vi "coke_can_current_version.vi"() -> ()   [LabVIEW 2012]
uses:
  X:/Lab/Labmembers/Lukas Gemar/Control 1.ctl
  <vilib>/DAQmx/write.llb/DAQmx Write (Digital Bool 1Line 1Point).vi
  <vilib>/Analysis/baseanly.llb/Mean (DBL).vi
  <vilib>/DAQmx/create/channels.llb/DAQmx Create Channel (DO-Digital Output).vi
  <vilib>/DAQmx/miscellaneous.llb/DAQmx Fill In Error Info.vi
  <vilib>/Analysis/NI_AALBase.lvlib
  Program Files/ALP-4.1/ALP-4.1 high-speed API/Samples/alpD41.dll
panel:
  in  "Bin (n x n) 2":u16(ring)=1 caption="Cursor Bin" items=["1x1"=1, "2x2"=2, "4x4"=4]
  in  "Tab Control":T1(tab)
  out "Initialize":u32
  out "Initialize?":bool
  out "Bits per Channel":i32
  out "camera initialization error":errorcluster
  out "Camera ID":string="0"
  out "Model":string="0"
  out "y pixels":i32
  out "x pixels":i32
  out "ROI cursor":T2={"x offset"=480, "y offset"=456, "x width"=68, "y width"=76} {"x offset" min=1 max=512 step=1; "y offset" min=1 max=512 step=1; "x width" min=1 max=512 step=1; "y width" min=1 max=512 step=1}
  out "Previous Bin":u16(ring)=2 caption="Cursor Bin" items=["1x1"=1, "2x2"=2, "4x4"=4]
  in  "473nm line":tag="Dev1/ao1"
  in  "635nm dig line":tag="Dev1/port0/line2"
  out "SerialNumber":i32
  out "DevAllocErr":i32
  out "DevInq1":errorcluster
  in  "Select Mov":bool
  in  "User Movie Path":path=path "C:/data/Lukas_data/movie.bin"
  in  "635nm":bool
  in  "All On":bool
  out "Movie Complete":bool caption="Movie Complete:"
  in  "Play Movie":bool
  in  "Make Movie":bool
  in  "Define Object":bool
  in  "Previous ROI 2":bool
  out "Previous ROI":T2={"x offset"=256, "y offset"=256, "x width"=512, "y width"=512} caption="Previous" {"x offset" min=1 max=512 step=1; "y offset" min=1 max=512 step=1; "x width" min=1 max=512 step=1; "y width" min=1 max=512 step=1}
  in  "Update ROI":bool
  in  "ROI":T2={"x offset"=960, "y offset"=912, "x width"=136, "y width"=152} caption="Current" {"x offset" min=1 max=2048 step=1; "y offset" min=1 max=2048 step=1; "x width" min=1 max=2048 step=1; "y width" min=1 max=2048 step=1}
  in  "Symmetrical":bool=TRUE
  in  "Draw ROI":bool
  in  "ROI selection":u16(ring) items=["Full ROI", "Central quad", "Red Laser ROI", "Custom ROI"]
  in  "Stop Program":bool
  in  "Enter Live Mode":bool
  out "Image":i32[][](graph)
  out "mean":dbl=701.2764784557547
  out "max value":u16=1056
  out "min value":u16=384
  out "Histogram":T3(graph)={"X Values"=[417.6, 484.8, 552.0, 619.2, 686.4, 753.6, 820.8, 888.0, 955.2, 1022.4], "Histogram: h(x)"=[403, 4234, 6440, 8496, 9541, 10568, 10361, 4568, 669, 48]}
  out "Camera Error":errorcluster
  out "Location indicator":u16[][](graph)
  in  "Clicky Movie Path":path=path "C:/data/Lukas_data/movie.bin"
  in  "Contrast\nAdjust":cluster{i32, i32}(slide) scale=100.0..65535.0
  in  "Register!":bool
  in  "Image Registration":bool
  out "Status":string="Ready"
  out "max frame rate (Hz)":dbl
  in  "Exposure (msec)":T4=100.0
  in  "base path":path=path "C:/data/Lukas_data"
  in  "File Name":string
  out "Frames Recorded":i32
  in  "Bin (n x n)":u16(ring)=1 caption="Cursor Bin" items=["1x1"=1, "2x2"=2, "4x4"=4]
  in  "Acquire movie":bool
  in  "# frames":u32=100
  out "Total time (sec)":dbl=100.0 min=1.0 max=5000.0 step=1.0
  out "Elapsed time (sec)":dbl=100.0 min=1.0 max=5000.0 step=1.0
  in  "Snap and Save":bool
  in  "Trigger":bool=TRUE
  in  "Color Box 2":u32(colorbox)=5470810
  in  "Color Box 3":u32(colorbox)=6118749
  in  "Color Box 4":u32(colorbox)
  in  "Color Box 5":u32(colorbox)
  in  "473nm":bool
  in  "473 signal":dbl=0.5 min=0.0 max=0.5
  in  "Color Box 6":u32(colorbox)
  out "# of Objects":dbl
  in  "Color Box":u32(colorbox)=6581130
  out "Matlab Error":errorcluster
  in  "Image Reg Path":path=path "C:/data/Lukas_data/image_reg.bin"
  out "DeviceID":u32
  out "SequID":u32
  in  "DMD_trigger":tag="Dev1/port0/line0" caption="DMD trigger"
  in  "DAQ Error":errorcluster
  in  "Image Reg ctl points":path=path "C:/data/Lukas_data/image_reg.txt"
  in  "Transformation path":path=path "C:/data/Lukas_data/transform.txt"
  out "DevFreeErr":i32
  out "SeqFreeErr":i32
  out "ALP_Error":errorcluster
  # "Camera initialization"
  # "Laser initialization"
  # "Extra Variables"
  # "DMD initialization"
  # "ROI Control"
  # "LIVE Mode Settings"
  # "external"
  # "internal"
  # "Object Control"
  # "Image Registration"
  # "Lasers"
  # "High"
  # "Low"
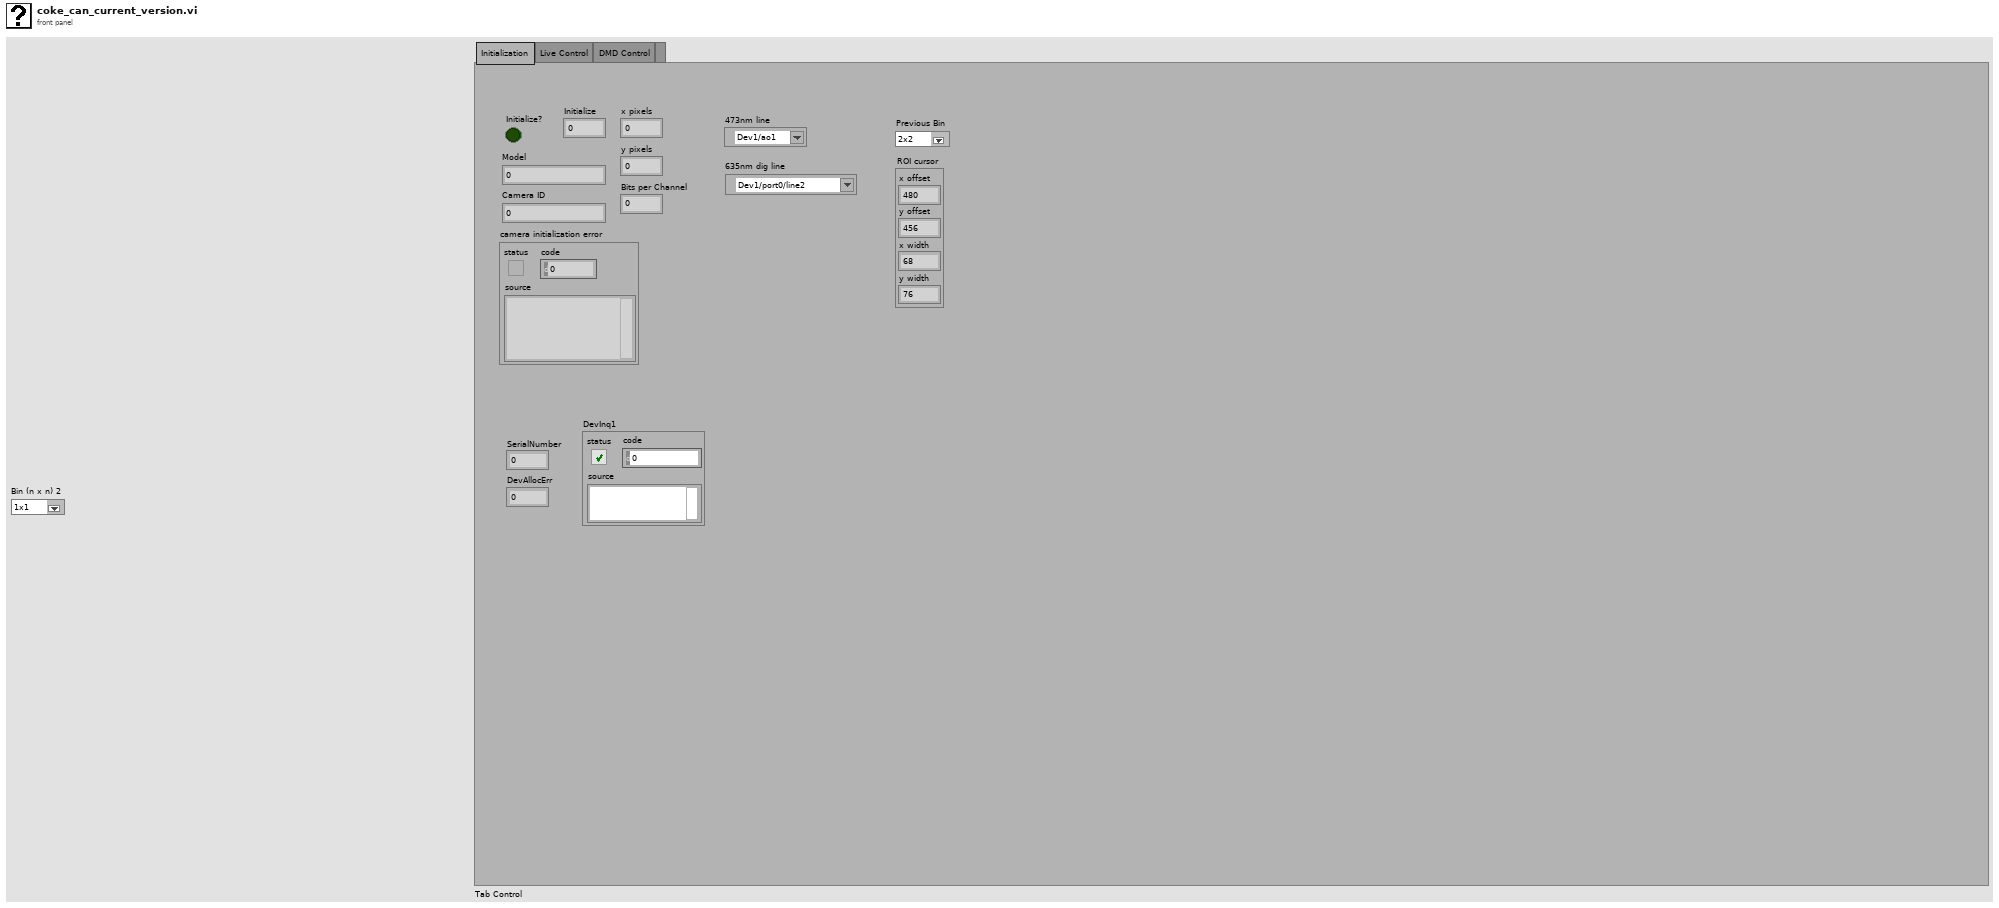
[diagram p1: front panel]
types:
  T1 = enum32{"Initialization", "Live Control", "DMD Control", ""}
  T2 = cluster{"x offset":i32, "y offset":i32, "x width":i32, "y width":i32}
  T3 = cluster{"X Values":dbl[], "Histogram: h(x)":i32[]}
  T4 = typedef "Control 1.ctl" = dbl
  T5 = enum8{"Enabled", "Disabled", "Disabled and Grayed Out"}
  T6 = cluster{"width":u32, "height":u32, "datatype":u32}
  T7 = cluster{"Horizontal Offset":i32, "Vertical Offset":i32, "Horizontal Width":i32, "Vertical Width":i32}
  T8 = cluster{"Value":i32, "Minimum":i32, "Maximum":i32, "Increment":i32}
  T9 = cluster{"X min":dbl, "Y min":dbl, "X max":dbl, "Y max":dbl}
  T10 = cluster{"Cursor.Cursor X":dbl, "Cursor.Cursor Y":dbl, "Cursor.Cursor X":dbl, "Cursor.Cursor Y":dbl}
  T11 = cluster{"Cursor1. X":dbl, "Cursor1. Y":dbl, "Cursor2. X":dbl, "Cursor2. Y":dbl}
  T12 = cluster{"x offset":dbl, "y offset":dbl, "x width":dbl, "y width":dbl}
  T13 = typedef "LVPointDoubleTypeDef.ctl" = cluster{"Cursor X":dbl, "Cursor Y":dbl}
  T14 = cluster{"XScale.Minimum":dbl, "YScale.Minimum":dbl, "XScale.Maximum":dbl, "YScale.Maximum":dbl}
  T15 = cluster{"Cursor.Cursor Position":T13, "Cursor.Cursor Position":T13}
  T16 = cluster{"Cursor1.Position":T13, "Cursor2.Position":T13}
  T17 = cluster{"Active Cursor":u32, "Active Cursor":u32, dbl, dbl}
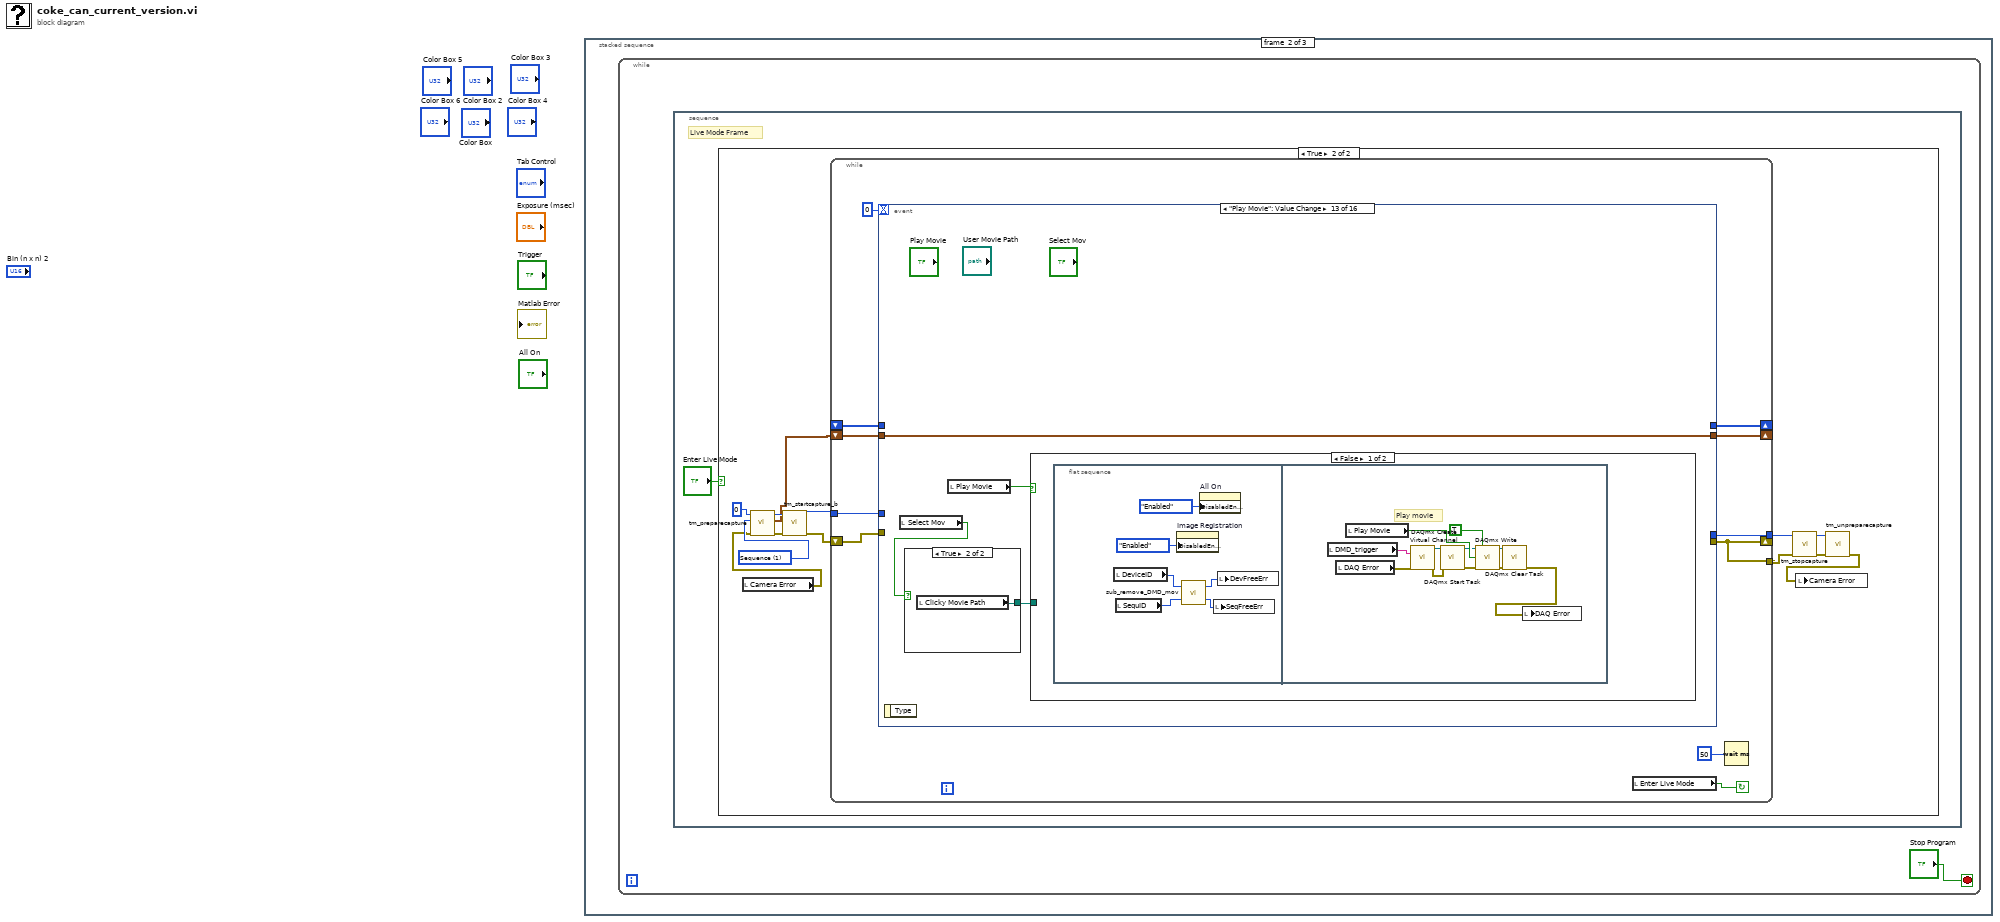
[diagram p0: block diagram]
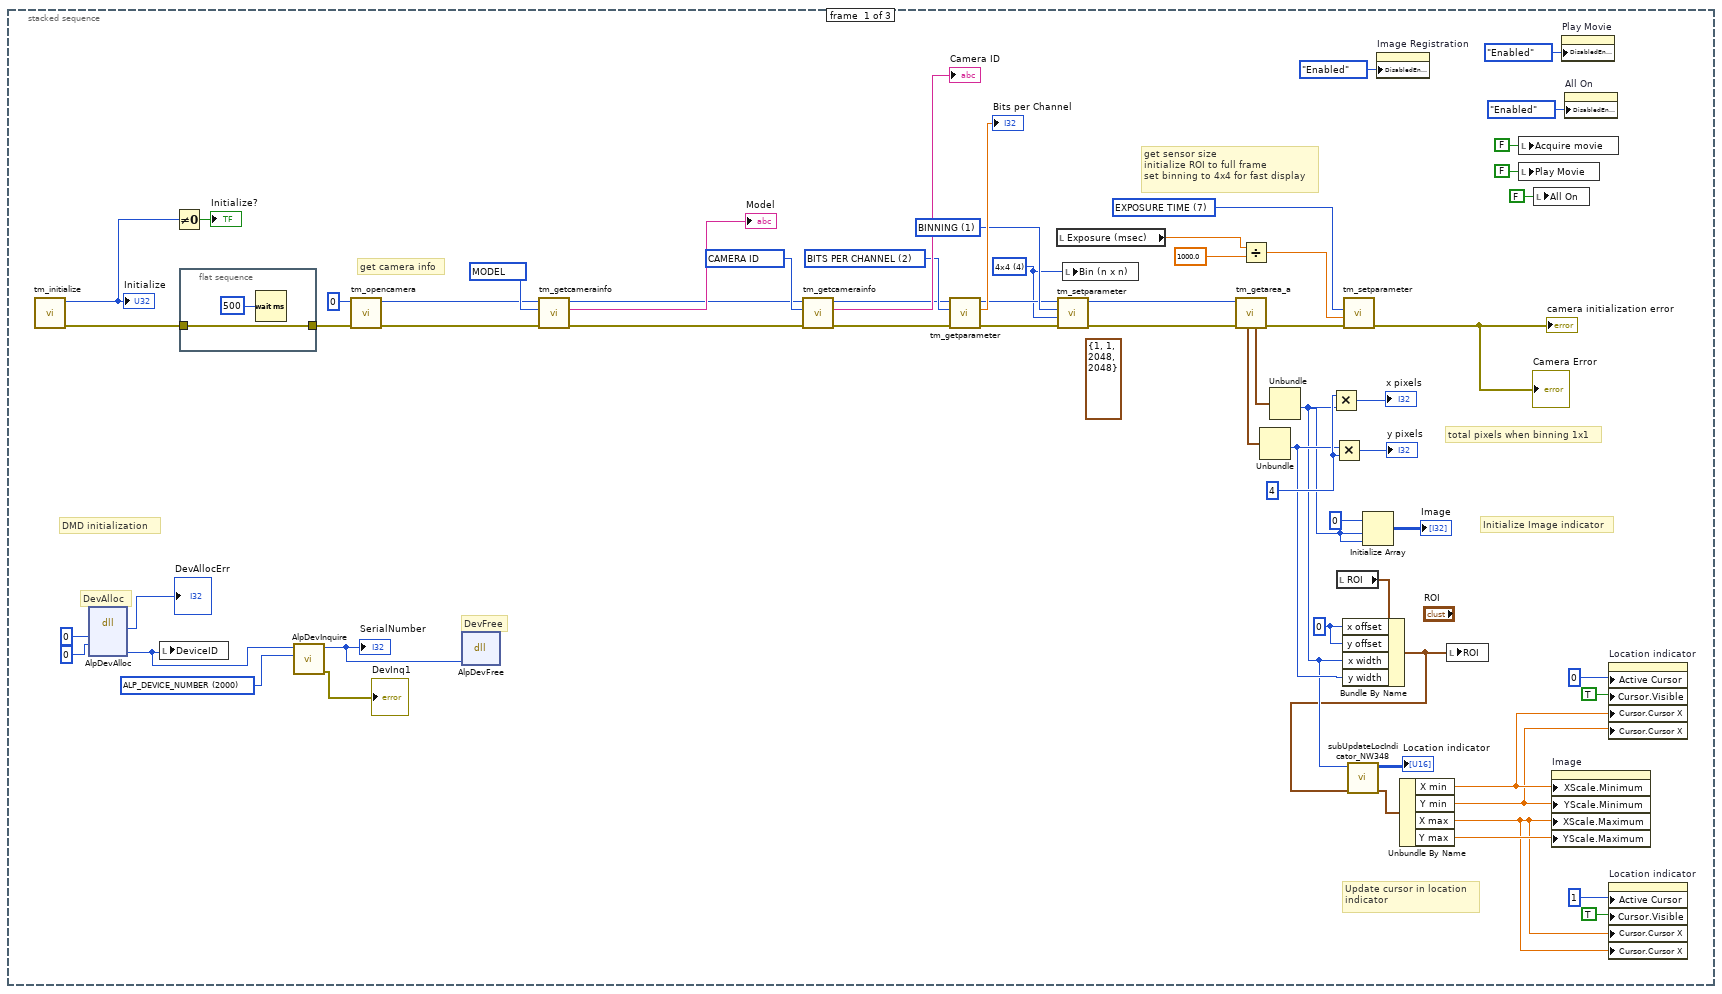
[diagram p2: hidden frame]
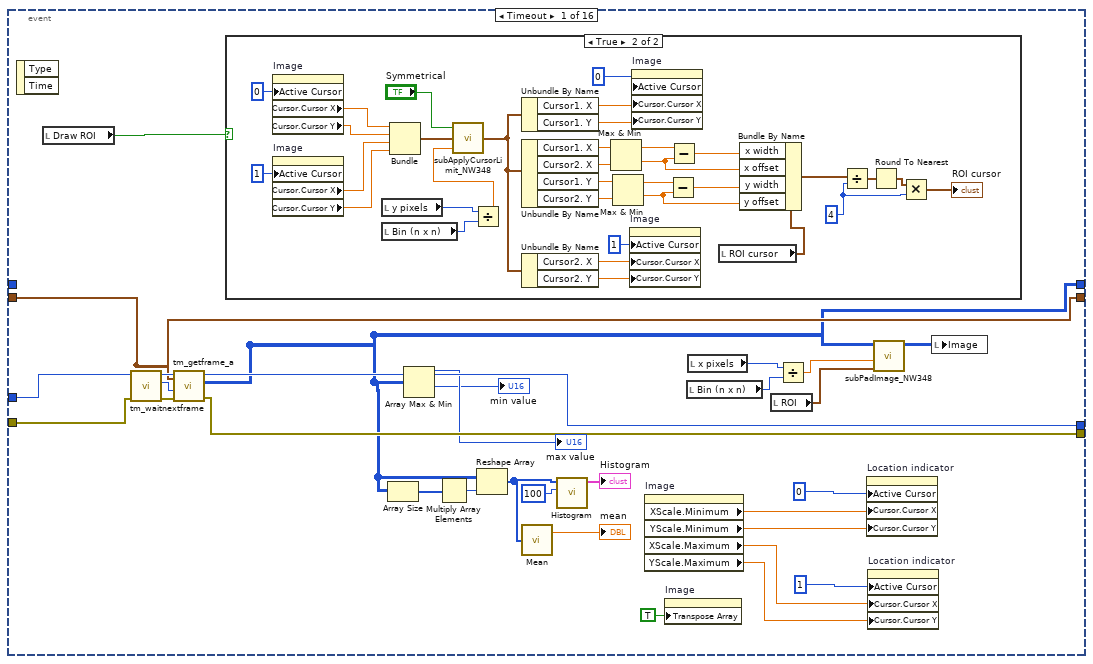
[diagram p4: hidden frame]
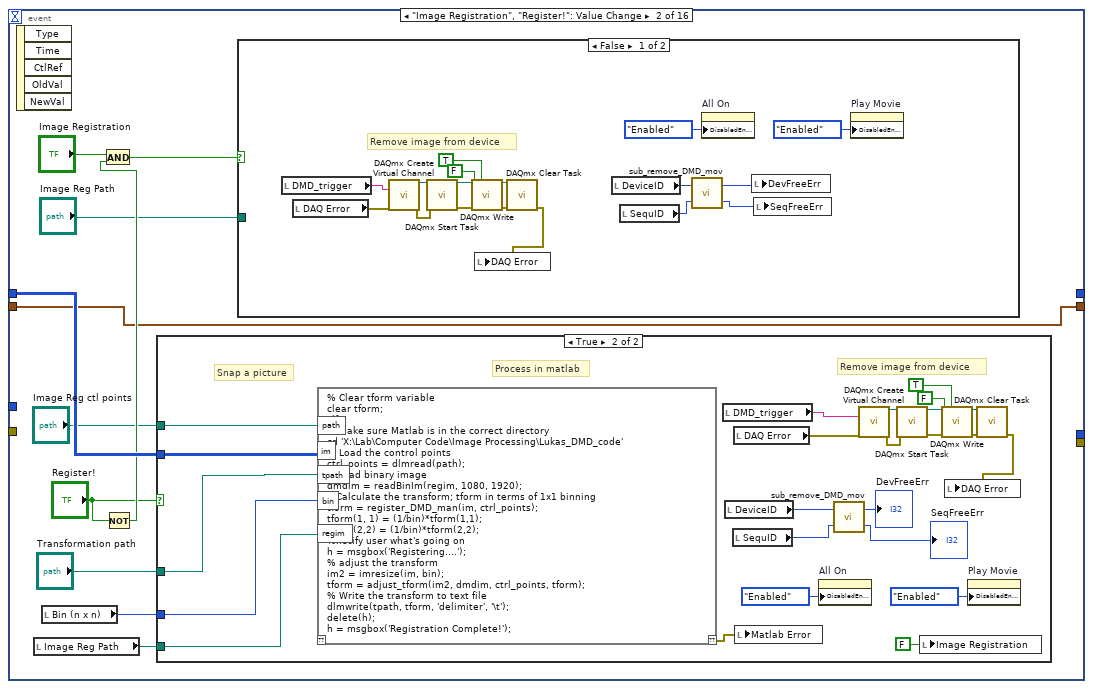
[diagram p6: hidden frame]
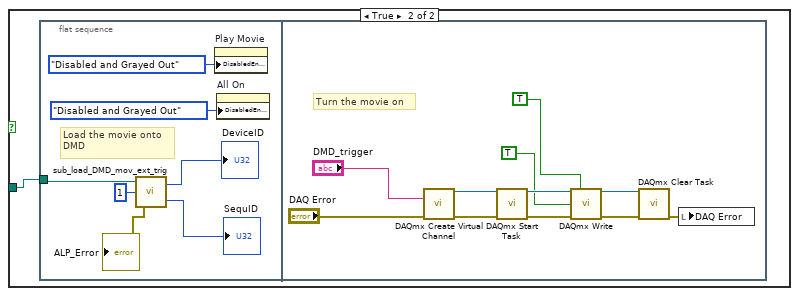
[diagram p8: hidden frame]
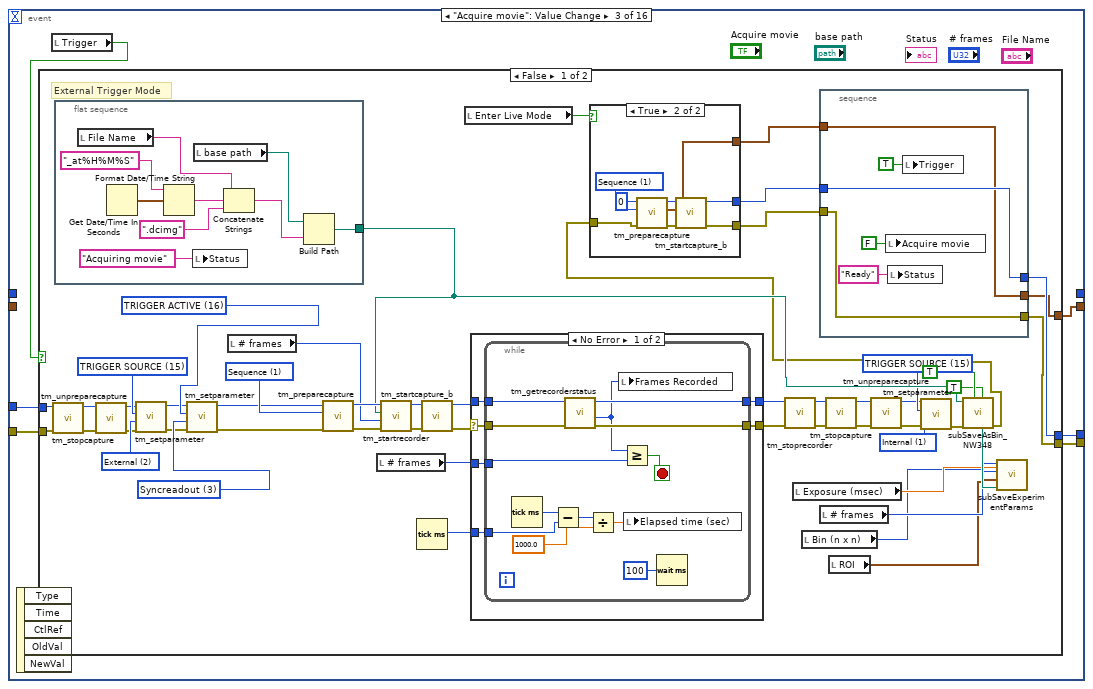
[diagram p9: hidden frame]
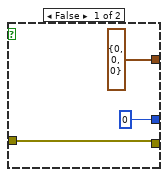
[diagram p10: hidden frame]
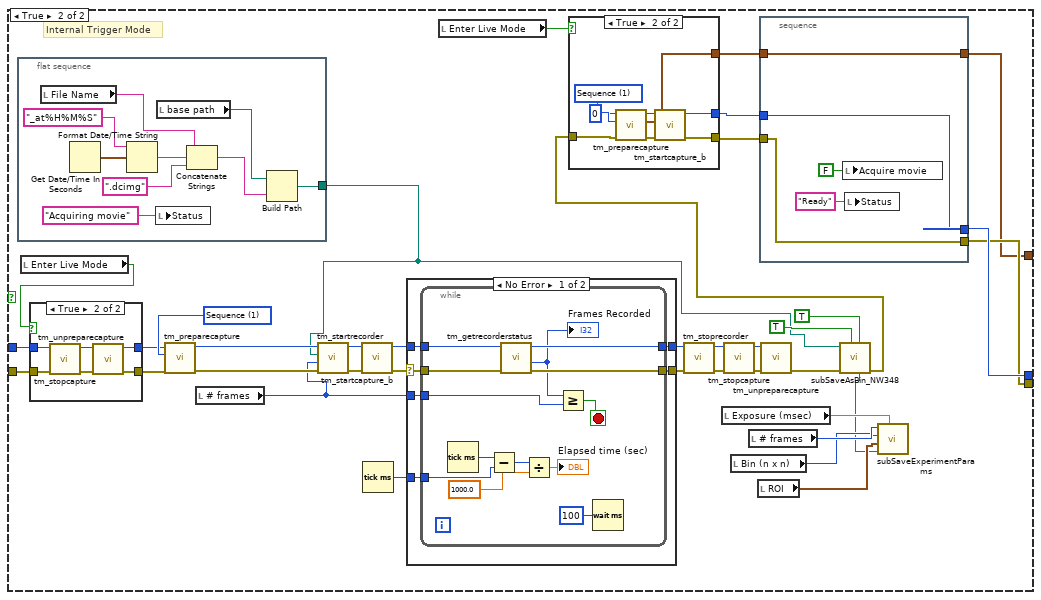
[diagram p12: hidden frame]
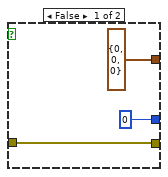
[diagram p13: hidden frame]
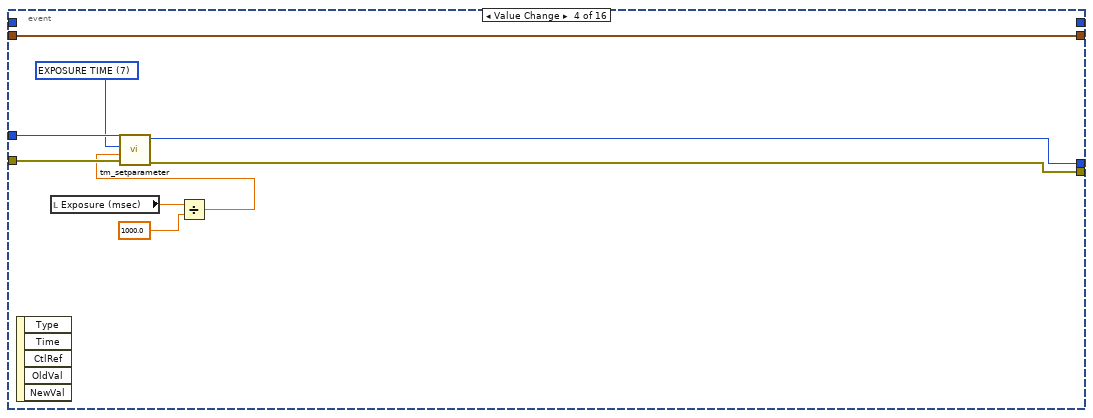
[diagram p16: hidden frame]
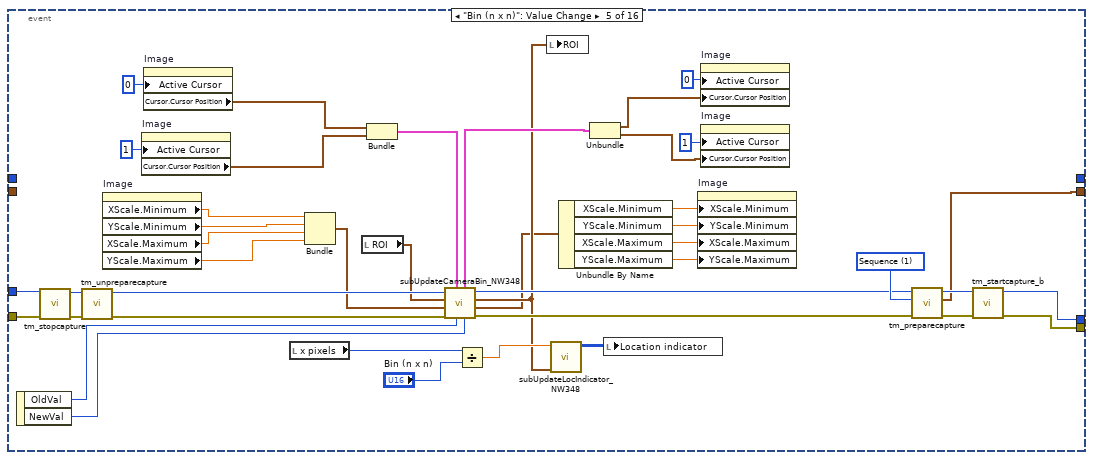
[diagram p17: hidden frame]
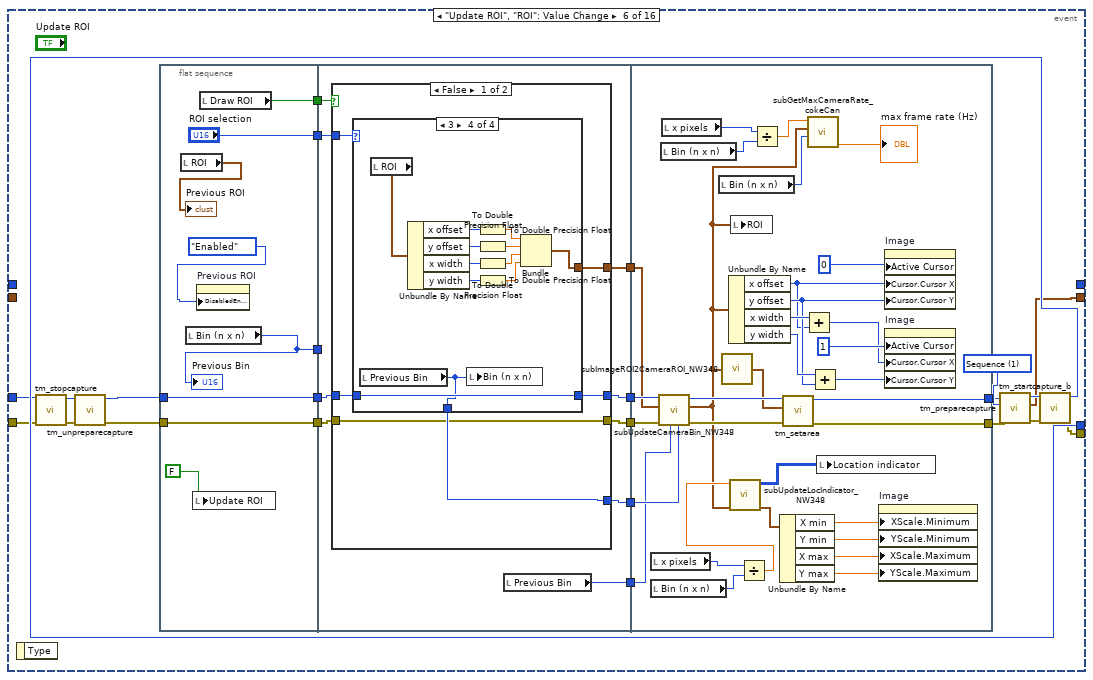
[diagram p18: hidden frame]
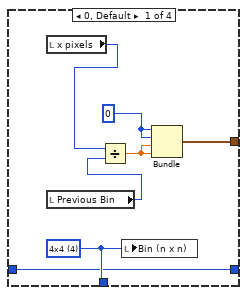
[diagram p19: hidden frame]
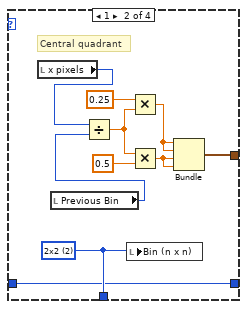
[diagram p20: hidden frame]
diagram:
  n1 = stacked-sequence {
    frame #0 {
      w5 = 2000 items=["ALP_DEVICE_NUMBER"=2000, "ALP_VERSION"=2001, "ALP_DEV_STATE"=2002, "ALP_AVAIL_MEMORY"=2003, "ALP_SYNCH_POLARITY"=2004, "ALP_TRIGGER_EDGE"=2005, "ALP_USB_CONNECTION"=2016, "ALP_DEV_DMDTYPE"=2021, "ALP_DEV_DISPLAY_HEIGHT"=2057, "ALP_DEV_DISPLAY_WIDTH"=2058, "ALP_PWM_LEVEL"=2063, "ALP_DEV_DMD_MODE"=2064] ("InquireType")
      w29 = 0 ("x offset")
      w41 = 4
      (unwired) T7 {"Horizontal Offset"=1, "Vertical Offset"=1, "Horizontal Width"=2048, "Vertical Width"=2048} ("Sub Region")
      w15 = u16 4 items=["1x1"=1, "2x2"=2, "4x4"=4] ("Bin (n x n)")
      w48 = 7 items=["BINNING"=1, "BITS PER CHANNEL"=2, "ACTIVE VIEW INDEX"=3, "CCD MODE"=4, "SENSOR MODE"=5, "READOUT MODE"=6, "EXPOSURE TIME"=7, "CONTRAST GAIN"=8, "CONTRAST OFFSET"=9, "LIGHT MODE"=10, "SENSITIVITY"=11, "WHITE BALANCE"=12, "PHOTON IMAGING MODE"=13, "HIGH DYNAMIC RANGE MODE"=14, "TRIGGER SOURCE"=15, "TRIGGER ACTIVE"=16, "TRIGGER MODE"=17, "TRIGGER POLARITY"=18, "TRIGGER GLOBAL EXPOSURE"=19, "FIRST TRIGGER BEHAVIOR"=20, "TRIGGER TIMES"=21, "OUTPUT TRIGGER POLARITY"=22, "OUTPUT TRIGGER DELAY"=23, "OUTPUT TRIGGER PERIOD"=24, "TEMPERATURE"=25, "TEMPERATURE TARGET"=26, "SENSOR COOLER FAN"=27, "MECHANICAL SHUTTER"=28, "BACK FOCUS POSITION"=29, "FRAMEBUNDLE MODE"=30, "FRAMEBUNDLE NUMBER"=31, "LINEBUNDLE HEIGHT"=32, "TRIGGER CONNECTOR"=33, "IMAGE PIXEL TYPE"=34] ("Parameter")
      w52 = 1 items=["BINNING"=1, "BITS PER CHANNEL"=2, "ACTIVE VIEW INDEX"=3, "CCD MODE"=4, "SENSOR MODE"=5, "READOUT MODE"=6, "EXPOSURE TIME"=7, "CONTRAST GAIN"=8, "CONTRAST OFFSET"=9, "LIGHT MODE"=10, "SENSITIVITY"=11, "WHITE BALANCE"=12, "PHOTON IMAGING MODE"=13, "HIGH DYNAMIC RANGE MODE"=14, "TRIGGER SOURCE"=15, "TRIGGER ACTIVE"=16, "TRIGGER MODE"=17, "TRIGGER POLARITY"=18, "TRIGGER GLOBAL EXPOSURE"=19, "FIRST TRIGGER BEHAVIOR"=20, "TRIGGER TIMES"=21, "OUTPUT TRIGGER POLARITY"=22, "OUTPUT TRIGGER DELAY"=23, "OUTPUT TRIGGER PERIOD"=24, "TEMPERATURE"=25, "TEMPERATURE TARGET"=26, "SENSOR COOLER FAN"=27, "MECHANICAL SHUTTER"=28, "BACK FOCUS POSITION"=29, "FRAMEBUNDLE MODE"=30, "FRAMEBUNDLE NUMBER"=31, "LINEBUNDLE HEIGHT"=32, "TRIGGER CONNECTOR"=33, "IMAGE PIXEL TYPE"=34] ("Parameter")
      w54 = 2 items=["BINNING"=1, "BITS PER CHANNEL"=2, "ACTIVE VIEW INDEX"=3, "CCD MODE"=4, "SENSOR MODE"=5, "READOUT MODE"=6, "EXPOSURE TIME"=7, "CONTRAST GAIN"=8, "CONTRAST OFFSET"=9, "LIGHT MODE"=10, "SENSITIVITY"=11, "WHITE BALANCE"=12, "PHOTON IMAGING MODE"=13, "HIGH DYNAMIC RANGE MODE"=14, "TRIGGER SOURCE"=15, "TRIGGER ACTIVE"=16, "TRIGGER MODE"=17, "TRIGGER POLARITY"=18, "TRIGGER GLOBAL EXPOSURE"=19, "FIRST TRIGGER BEHAVIOR"=20, "TRIGGER TIMES"=21, "OUTPUT TRIGGER POLARITY"=22, "OUTPUT TRIGGER DELAY"=23, "OUTPUT TRIGGER PERIOD"=24, "TEMPERATURE"=25, "TEMPERATURE TARGET"=26, "SENSOR COOLER FAN"=27, "MECHANICAL SHUTTER"=28, "BACK FOCUS POSITION"=29, "FRAMEBUNDLE MODE"=30, "FRAMEBUNDLE NUMBER"=31, "LINEBUNDLE HEIGHT"=32, "TRIGGER CONNECTOR"=33, "IMAGE PIXEL TYPE"=34] ("Parameter")
      w58 = u32 67109122 items=["BUS"=67109121, "CAMERA ID"=67109122, "VENDOR"=67109123, "MODEL"=67109124, "CAMERA VERSION"=67109125, "DRIVER VERSION"=67109126, "MODULE VERSIOIN"=67109127, "DCAMAPI VERSION"=67109128] ("Info ID")
      w57 = u32 67109124 items=["BUS"=67109121, "CAMERA ID"=67109122, "VENDOR"=67109123, "MODEL"=67109124, "CAMERA VERSION"=67109125, "DRIVER VERSION"=67109126, "MODULE VERSIOIN"=67109127, "DCAMAPI VERSION"=67109128] ("Info ID")
      # "DMD initialization"
      # "DevFree"
      # "DevAlloc"
      # "Update cursor in location\nindicator"
      # "total pixels when binning 1x1"
      # "Initialize Image indicator"
      # "get sensor size\ninitialize ROI to full frame\nset binning to 4x4 for fast display"
      # "get camera info"
      n2 = call <userlib>:"tm_initialize.vi"() -> ("error out"=w51:errorcluster, "Number Of Cameras"=w62:u32)  [unwired: 10 in]
      "Initialize" <- w62
      n3 = dll-call lib="C:/Program Files/ALP-4.1/ALP-4.1 high-speed API/Samples/alpD41.dll" fn="AlpDevAlloc"("DeviceNum"=0, "InitFlag"=0) -> ("return type"=→"DevAllocErr":i32, "DeviceIdPtr"=w4:u32)  [unwired: 6 in, 2 out]
      n4 = local write "DeviceID"(w4) -> ()
      n5 = Not Equal To 0?(x=w62) -> (x != 0?=→"Initialize?":bool)
      n6 = flat-sequence {
        tunnel: w51 -> [w65]
        tunnel: [w65] -> w50
        frame #0 {
          n7 = Wait (ms)(milliseconds to wait=u32 500) -> ()  [unwired: 1 out]
        }
      }
      n8 = call "AlpDevInquire.vi"("InquireType"=w5, "DeviceID"=w4) -> ("Error OUT"=→"DevInq1":errorcluster, "DeviceIDout"=w2:u32)  [unwired: 6 in, 2 out]
      "SerialNumber" <- w2
      n9 = call <userlib>:"tm_opencamera.vi"("error in (no error)"=w50, "Camera Index"=u32 0 ("milliseconds to wait")) -> ("error out"=w60:errorcluster, "Handle out"=w38:u32)  [unwired: 8 in]
      n10 = dll-call lib="C:/Program Files/ALP-4.1/ALP-4.1 high-speed API/Samples/alpD41.dll" fn="AlpDevFree"("DeviceId"=w2) -> ()  [unwired: 5 in, 2 out]
      n11 = call <userlib>:"tm_getcamerainfo.vi"("error in (no error)"=w60, "Info ID"=w57, "Handle in"=w38) -> ("error out"=w56:errorcluster, "String"=→"Model":string, "Handle out"=w37:u32)  [unwired: 6 in]
      n12 = call <userlib>:"tm_getcamerainfo.vi"("error in (no error)"=w56, "Info ID"=w58, "Handle in"=w37) -> ("error out"=w45:errorcluster, "String"=→"Camera ID":string, "Handle out"=w36:u32)  [unwired: 6 in]
      n13 = call <userlib>:"tm_getparameter.vi"("error in (no error)"=w45, "Parameter"=w54, "Handle in"=w36) -> ("error out"=w47:errorcluster, "Value out"=→"Bits per Channel":dbl, "Handle out"=w35:u32)  [unwired: 6 in]
      n14 = local read "Exposure (msec)"() -> (w34:T4)
      n15 = call <userlib>:"tm_setparameter.vi"("error in (no error)"=w47, "Value in"=w15, "Parameter"=w52, "Handle in"=w35) -> ("error out"=w23:errorcluster, "Handle out"=w24:u32)  [unwired: 6 in]
      n16 = local write "Bin (n x n)"(w15) -> ()
      n17 = call <userlib>:"tm_getarea_a.vi"("error in (no error)"=w23, "Handle in"=w24) -> ("error out"=w49:errorcluster, "H Width"=w43:T8, "V Width"=w42:T8)  [unwired: 4 in, 3 out]
      n18 = Divide(x=w34, y=1000.0) -> (x/y=w63:T4)
      n19 = Unbundle(w42) -> ("Maximum"=w30:i32)  [unwired: 3 out]
      n20 = Unbundle(w43) -> ("Maximum"=w28:i32)  [unwired: 3 out]
      n21 = Multiply(x=w41, y=w28) -> (x*y=→"x pixels":i32)
      n22 = Multiply(x=w30, y=w41) -> (x*y=→"y pixels":i32)
      n23 = local read "ROI"() -> (w31:T2)
      n24 = Bundle By Name(cluster=w31, "x offset"=w29, "y offset"=w29, "x width"=w28, "y width"=w30) -> (w14:T2)
      n25 = call <userlib>:"tm_setparameter.vi"("error in (no error)"=w49, "Value in"=w63, "Parameter"=w48) -> ("error out"=→"camera initialization error" →"Camera Error":errorcluster)  [unwired: 7 in, 1 out]
      n26 = call "subUpdateLocIndicator_NW348.vi"("ROI"=w14, "pixel range"=w28) -> ("Graph scale"=w27:T9, "Location indicator"=→"Location indicator":u16[][])  [unwired: 8 in]
      n27 = Initialize Array(0, w28, w28) -> (→"Image":i32[][])
      n28 = property on="Image Registration" class="Bool (strict)"("DisabledEnum"=T5."Enabled" ("Disabled")) -> ()  [unwired: 2 in, 2 out]
      n29 = Unbundle By Name(w27) -> ("X min"=w20:dbl, "Y min"=w19:dbl, "X max"=w16:dbl, "Y max"=w26:dbl)
      n30 = local write "ROI"(w14) -> ()
      n31 = local write "Acquire movie"(FALSE ("Acquire movie")) -> ()
      n32 = local write "Play Movie"(FALSE ("Play Movie")) -> ()
      n33 = local write "All On"(FALSE ("All On")) -> ()
      n34 = property on="Image" class="IntGraph (strict)"("XScale.Minimum"=w20, "YScale.Minimum"=w19, "XScale.Maximum"=w16, "YScale.Maximum"=w26) -> ()  [unwired: 2 in, 2 out]
      n35 = property on="Play Movie" class="Bool (strict)"("DisabledEnum"=T5."Enabled" ("Disabled")) -> ()  [unwired: 2 in, 2 out]
      n36 = property on="All On" class="Bool (strict)"("DisabledEnum"=T5."Enabled" ("Disabled")) -> ()  [unwired: 2 in, 2 out]
      n37 = property on="Location indicator" class="IntGraph (strict)"("Active Cursor"=0 ("x offset"), "Cursor.Visible"=TRUE, "Cursor.Cursor X"=w20, "Cursor.Cursor X"=w19) -> ()  [unwired: 2 in, 2 out]
      n38 = property on="Location indicator" class="IntGraph (strict)"("Active Cursor"=1 ("x offset"), "Cursor.Visible"=TRUE, "Cursor.Cursor X"=w16, "Cursor.Cursor X"=w16) -> ()  [unwired: 2 in, 2 out]
    }
    frame #1 {
      n39 = while {
        stop <- "Stop Program" stop-if-true
        n40 = stacked-sequence {
          frame #0 {
            # "Live Mode Frame"
            n41 = case shown="True" "Enter Live Mode" {
              frame False {
              }
              frame True {
                w81 = 1 items=["Snap", "Sequence"] ("Capture mode")
                n42 = local read "Camera Error"() -> (w70:errorcluster)
                n43 = call <userlib>:"tm_preparecapture.vi"("error in (no error)"=w70, "Capture mode"=w81, "Handle in"=u32 0) -> ("error out"=w79:errorcluster, "Buffer"=w69:T6, "Handle out"=w80:u32)  [unwired: 5 in, 1 out]
                n44 = call <userlib>:"tm_startcapture_b.vi"("error in (no error)"=w79, "Handle in"=w80) -> ("error out"=w77:errorcluster, "Handle out"=w76:u32)  [unwired: 8 in]
                n45 = while {
                  tunnel: [w91] -> w72
                  shift-right: [w88] -> _
                  shift-left: w77 -> [w90]
                  tunnel: w76 -> [w89]
                  tunnel: [w88] -> w73
                  shift-right: [w85] -> _
                  shift-left: _ -> [w84]
                  shift-right: [w83] -> _
                  shift-left: w69 -> [w82]
                  stop <- w92 continue-if-true
                  n46 = event shown="[12] \"Play Movie\": Value Change" {
                    selector: _ -> [_ _ _ _ _ _ _ _ _ _ _ _ _ _ _ _]
                    dyn-events: _ -> [_ _ _ _ _ _ _ _ _ _ _ _ _ _ _ _]
                    timeout: 0 -> [_ _ _ _ _ _ _ _ _ _ _ _ _ _ _ _]
                    tunnel: [w122 _ w231 w429 w441 w487 w605 w626 _ w668 w696 _ _ w753 w778 _] -> w91
                    tunnel: w90 -> [w121 _ w233 w427 w472 w479 w604 w619 _ w669 w695 _ _ w752 w777 _]
                    tunnel: w89 -> [w120 _ w232 w431 w473 w478 w605 w620 _ w668 w696 _ _ w753 w778 _]
                    tunnel: [w119 _ w230 w428 w440 w486 w604 w625 _ w669 w695 _ _ w752 w777 _] -> w88
                    tunnel: [w93 _ _ _ _ _ _ _ _ _ _ _ _ _ _ _] -> w85
                    tunnel: w84 -> [_ w167 _ _ _ _ _ _ _ w667 w699 _ _ _ _ _]
                    tunnel: [w95 w159 w228 w423 w444 w485 w603 w618 w656 w665 w702 w704 w712 w751 w779 w780] -> w83
                    tunnel: w82 -> [w95 w159 _ w423 _ _ w603 _ w656 w665 w702 w704 w712 w751 w779 w780]
                    event Timeout {
                      n47 = event-data() -> ()  [unwired: 1 in, 2 out]
                      n48 = local read "Draw ROI"() -> (w109:bool)
                      n49 = call <userlib>:"tm_waitnextframe.vi"("error in (no error)"=w121, "Handle in"=w120) -> ("error out"=w111:errorcluster, "Frame Index"=w113:i32, "Handle out"=w112:u32)  [unwired: 6 in, 1 out]
                      n50 = call <userlib>:"tm_getframe_a.vi"("error in (no error)"=w111, "Frame Index"=w113, "Buffer"=w95, "Handle in"=w112) -> ("error out"=w119:errorcluster, "Data 16"=w93:u16[][], "Handle out"=w122:u32)  [unwired: 4 in, 1 out]
                      n51 = case shown="True" w109 {
                        frame False {
                        }
                        frame True {
                          w124 = u32 4 ("Active Cursor")
                          n52 = property on="Image" class="IntGraph (strict)"("Active Cursor"=u32 0) -> ("Cursor.Cursor X"=w152:dbl, "Cursor.Cursor Y"=w151:dbl)  [unwired: 2 in, 2 out]
                          n53 = property on="Image" class="IntGraph (strict)"("Active Cursor"=u32 1) -> ("Cursor.Cursor X"=w154:dbl, "Cursor.Cursor Y"=w153:dbl)  [unwired: 2 in, 2 out]
                          n54 = local read "y pixels"() -> (w147:i32)
                          n55 = local read "Bin (n x n)"() -> (w148:u16)
                          n56 = Bundle("Cursor.Cursor X"=w152, "Cursor.Cursor Y"=w151, "Cursor.Cursor X"=w154, "Cursor.Cursor Y"=w153) -> (w150:T10)  [unwired: 1 in]
                          n57 = Divide(x=w147, y=w148) -> (x/y=w146:dbl)
                          n58 = call "subApplyCursorLimit_NW348.vi"("Cursor limit"=w146, "Cursor input"=w150, "Symmetrical ROI"="Symmetrical") -> ("Cursor output"=w145:T11)  [unwired: 2 in]
                          n59 = Unbundle By Name(w145) -> ("Cursor1. X"=w143:dbl, "Cursor1. Y"=w142:dbl)
                          n60 = Unbundle By Name(w145) -> ("Cursor1. X"=w138:dbl, "Cursor2. X"=w137:dbl, "Cursor1. Y"=w135:dbl, "Cursor2. Y"=w136:dbl)
                          n61 = Unbundle By Name(w145) -> ("Cursor2. X"=w140:dbl, "Cursor2. Y"=w139:dbl)
                          n62 = Max & Min(x=w138, y=w137) -> (max(x,y)=w134:dbl, min(x,y)=w132:dbl)
                          n63 = Max & Min(x=w135, y=w136) -> (max(x,y)=w133:dbl, min(x,y)=w129:dbl)
                          n64 = property on="Image" class="IntGraph (strict)"("Active Cursor"=u32 1, "Cursor.Cursor X"=w140, "Cursor.Cursor Y"=w139) -> ()  [unwired: 2 in, 2 out]
                          n65 = property on="Image" class="IntGraph (strict)"("Active Cursor"=u32 0, "Cursor.Cursor X"=w143, "Cursor.Cursor Y"=w142) -> ()  [unwired: 2 in, 2 out]
                          n66 = Subtract(x=w133, y=w129) -> (x-y=w130:dbl)
                          n67 = Subtract(x=w134, y=w132) -> (x-y=w131:dbl)
                          n68 = local read "ROI cursor"() -> (w128:T2)
                          n69 = Bundle By Name(cluster=w128, "x width"=w131, "x offset"=w132, "y width"=w130, "y offset"=w129) -> (w127:T2)
                          n70 = Divide(x=w127, y=w124) -> (x/y=w126:T12)
                          n71 = Round To Nearest(number=w126) -> (nearest integer value=w125:T12)
                          n72 = Multiply(x=w125, y=w124) -> (x*y=→"ROI cursor":T12)
                        }
                      }
                      n73 = Array Size(array=w93) -> (size(s)=w96:i32[])
                      n74 = Array Max & Min(array=w93) -> (max value=→"max value":u16, min value=→"min value":u16)  [unwired: 2 out]
                      n75 = Multiply Array Elements(1:w96) -> (0:w97:i32)
                      n76 = Reshape Array(w93, w97) -> (w118:u16[])
                      n77 = call-poly <vilib>:"Mean.vi"("X"=w118) -> ("mean"=→"mean":dbl)  [unwired: 1 out]
                      n78 = call <vilib>:"Histogram.vi"("intervals"=100, "X"=w118) -> ("Histogram Graph"=→"Histogram":T3)  [unwired: 6 in, 3 out]
                      n79 = property on="Image" class="IntGraph (strict)"() -> ("XScale.Minimum"=w106:dbl, "YScale.Minimum"=w105:dbl, "XScale.Maximum"=w104:dbl, "YScale.Maximum"=w103:dbl)  [unwired: 2 in, 2 out]
                      n80 = property on="Image" class="IntGraph (strict)"("Transpose Array"=TRUE) -> ()  [unwired: 2 in, 2 out]
                      n81 = local read "Bin (n x n)"() -> (w100:u16)
                      n82 = local read "x pixels"() -> (w101:i32)
                      n83 = local read "ROI"() -> (w98:T2)
                      n84 = Divide(x=w101, y=w100) -> (x/y=w99:dbl)
                      n85 = property on="Location indicator" class="IntGraph (strict)"("Active Cursor"=0 ("x offset"), "Cursor.Cursor X"=w106, "Cursor.Cursor Y"=w105) -> ()  [unwired: 2 in, 2 out]
                      n86 = property on="Location indicator" class="IntGraph (strict)"("Active Cursor"=1 ("x offset"), "Cursor.Cursor X"=w104, "Cursor.Cursor Y"=w103) -> ()  [unwired: 2 in, 2 out]
                      n87 = call "subPadImage_NW348.vi"("ROI"=w98, "Full size"=w99, "Image in"=w93) -> ("Image out"=w102:u16[][])  [unwired: 7 in, 1 out]
                      n88 = local write "Image"(w102) -> ()
                    }
                    event "Image Registration", "Register!": Value Change {
                      n89 = event-data() -> ()  [unwired: 1 in, 5 out]
                      n90 = local read "Image Reg Path"() -> (w157:path)
                      n91 = local read "Bin (n x n)"() -> (w158:u16)
                      n92 = Not(x="Register!") -> (.not. x?=w165:bool)
                      n93 = And(x="Image Registration", y=w165) -> (x .and. y?=w164:bool)
                      n94 = case shown="True" "Register!" {
                        tunnel: w167 -> [_ w191]
                        tunnel: "Image Reg ctl points" -> [_ w190]
                        tunnel: "Transformation path" -> [_ w189]
                        tunnel: w158 -> [_ w172]
                        tunnel: w157 -> [_ w170]
                        frame False {
                        }
                        frame True {
                          # "Remove image from device"
                          # "Process in matlab"
                          # "Snap a picture"
                          n95 = script code="% Clear tform variable\nclear tform;\nclf;  \n% Make sure Matlab is in the correct directory\ncd 'X:\\Lab\\Computer Code\\Image Processing\\Lukas_DMD_code'\n% Load the control points\nctrl_points = dlmread(path);  \n% read binary image\ndmdim = readBinIm(regim, 1080, 1920); \n%Calculate the transform; tform in terms of 1x1 binning\ntform = register_DMD_man(im, ctrl_points); \ntform(1, 1) = (1/bin)*tform(1,1); \ntform(2,2) = (1/bin)*tform(2,2); \n%notify user what's going on \nh = msgbox('Registering....'); \n% adjust the transform\nim2 = imresize(im, bin); \ntform = adjust_tform(im2, dmdim, ctrl_points, tform); \n% Write the transform to text file\ndlmwrite(tpath, tform, 'delimiter', '\\t'); \ndelete(h); \nh = msgbox('Registration Complete!');"("path"=w190, "im"=w191, "tpath"=w189, "bin"=w172, "regim"=w170) -> ("??"=w171:errorcluster)  [unwired: 1 in]
                          n96 = local read "DMD_trigger"() -> (w187:tag)
                          n97 = local read "DeviceID"() -> (w177:u32)
                          n98 = local read "SequID"() -> (w176:u32)
                          n99 = local read "DAQ Error"() -> (w188:errorcluster)
                          n100 = local write "Matlab Error"(w171) -> ()
                          n101 = property on="All On" class="Bool (strict)"("DisabledEnum"=T5."Enabled" ("Disabled")) -> ()  [unwired: 2 in, 2 out]
                          n102 = call "sub_remove_DMD_mov.vi"("SequenceId"=w176, "DeviceId"=w177) -> ("SeqFreeErr"=→"SeqFreeErr":i32, "DevFreeErr"=→"DevFreeErr":i32)
                          n103 = call-poly <vilib>:"DAQmx Create Virtual Channel.vi"("lines"=w187, "error in"=w188) -> ("task out"=w186:refnum<k21>, "error out"=w185:errorcluster)  [unwired: 3 in, 9 out]
                          n104 = call <vilib>:"DAQmx Start Task.vi"("task/channels in"=w186, "error in"=w185) -> ("task out"=w184:refnum<k21>, "error out"=w183:errorcluster)  [unwired: 12 out]
                          n105 = local write "Image Registration"(FALSE ("Image Registration")) -> ()
                          n106 = call-poly <vilib>:"DAQmx Write.vi"("task/channels in"=w184, "auto start"=TRUE, "data"=FALSE, "error in"=w183) -> ("task out"=w181:refnum<k21>, "error out"=w180:errorcluster)  [unwired: 9 in, 1 out]
                          n107 = property on="Play Movie" class="Bool (strict)"("DisabledEnum"=T5."Enabled" ("Disabled")) -> ()  [unwired: 2 in, 2 out]
                          n108 = call <vilib>:"DAQmx Clear Task.vi"("task in"=w181, "error in"=w180) -> ("error out"=w179:errorcluster)  [unwired: 13 out]
                          n109 = local write "DAQ Error"(w179) -> ()
                        }
                      }
                      n110 = case shown="False" w164 {
                        tunnel: "Image Reg Path" -> [_ w209]
                        frame False {
                          # "Remove image from device"
                          n111 = local read "DMD_trigger"() -> (w199:tag)
                          n112 = local read "DAQ Error"() -> (w198:errorcluster)
                          n113 = call-poly <vilib>:"DAQmx Create Virtual Channel.vi"("lines"=w199, "error in"=w198) -> ("task out"=w200:refnum<k21>, "error out"=w201:errorcluster)  [unwired: 3 in, 9 out]
                          n114 = call <vilib>:"DAQmx Start Task.vi"("task/channels in"=w200, "error in"=w201) -> ("task out"=w202:refnum<k21>, "error out"=w203:errorcluster)  [unwired: 12 out]
                          n115 = call-poly <vilib>:"DAQmx Write.vi"("task/channels in"=w202, "auto start"=TRUE, "data"=FALSE, "error in"=w203) -> ("task out"=w205:refnum<k21>, "error out"=w206:errorcluster)  [unwired: 9 in, 1 out]
                          n116 = call <vilib>:"DAQmx Clear Task.vi"("task in"=w205, "error in"=w206) -> ("error out"=w207:errorcluster)  [unwired: 13 out]
                          n117 = local write "DAQ Error"(w207) -> ()
                          n118 = local read "DeviceID"() -> (w196:u32)
                          n119 = local read "SequID"() -> (w197:u32)
                          n120 = call "sub_remove_DMD_mov.vi"("SequenceId"=w197, "DeviceId"=w196) -> ("SeqFreeErr"=w195:i32, "DevFreeErr"=w194:i32)
                          n121 = property on="All On" class="Bool (strict)"("DisabledEnum"=T5."Enabled" ("Disabled")) -> ()  [unwired: 2 in, 2 out]
                          n122 = local write "DevFreeErr"(w194) -> ()
                          n123 = local write "SeqFreeErr"(w195) -> ()
                          n124 = property on="Play Movie" class="Bool (strict)"("DisabledEnum"=T5."Enabled" ("Disabled")) -> ()  [unwired: 2 in, 2 out]
                        }
                        frame True {
                          n125 = flat-sequence {
                            tunnel: w209 -> [w216]
                            frame #0 {
                              # "Load the movie onto\nDMD"
                              n126 = call "sub_load_DMD_mov_ext_trig.vi"("SequenceRepeats"=1, "binary mov path"=w216) -> ("SequID"=→"SequID":u32, "DeviceID"=→"DeviceID":u32, "DevInq1"=→"ALP_Error":errorcluster)
                              n127 = property on="Play Movie" class="Bool (strict)"("DisabledEnum"=T5."Disabled and Grayed Out" ("Disabled")) -> ()  [unwired: 2 in, 2 out]
                              n128 = property on="All On" class="Bool (strict)"("DisabledEnum"=T5."Disabled and Grayed Out" ("Disabled")) -> ()  [unwired: 2 in, 2 out]
                            }
                            frame #1 {
                              # "Turn the movie on"
                              n129 = call-poly <vilib>:"DAQmx Create Virtual Channel.vi"("lines"="DMD_trigger", "error in"="DAQ Error") -> ("task out"=w222:refnum<k21>, "error out"=w223:errorcluster)  [unwired: 3 in, 9 out]
                              n130 = call <vilib>:"DAQmx Start Task.vi"("task/channels in"=w222, "error in"=w223) -> ("task out"=w224:refnum<k21>, "error out"=w227:errorcluster)  [unwired: 12 out]
                              n131 = call-poly <vilib>:"DAQmx Write.vi"("task/channels in"=w224, "auto start"=TRUE, "data"=TRUE, "error in"=w227) -> ("task out"=w225:refnum<k21>, "error out"=w226:errorcluster)  [unwired: 9 in, 1 out]
                              n132 = call <vilib>:"DAQmx Clear Task.vi"("task in"=w225, "error in"=w226) -> ("error out"=w217:errorcluster)  [unwired: 13 out]
                              n133 = local write "DAQ Error"(w217) -> ()
                            }
                          }
                        }
                      }
                    }
                    event "Acquire movie": Value Change {
                      n134 = event-data() -> ()  [unwired: 1 in, 5 out]
                      n135 = local read "Trigger"() -> (w229:bool)
                      n136 = case shown="False" w229 {
                        tunnel: w233 -> [w240 w368]
                        tunnel: w232 -> [w239 w367]
                        tunnel: [w254 w341] -> w231
                        tunnel: [w250 w340] -> w230
                        tunnel: [w253 w337] -> w228
                        frame False {
                          w237 = 1 items=["Internal"=1, "External"=2, "Software"=3] ("Trigger Source")
                          w238 = 15 items=["BINNING"=1, "BITS PER CHANNEL"=2, "ACTIVE VIEW INDEX"=3, "CCD MODE"=4, "SENSOR MODE"=5, "READOUT MODE"=6, "EXPOSURE TIME"=7, "CONTRAST GAIN"=8, "CONTRAST OFFSET"=9, "LIGHT MODE"=10, "SENSITIVITY"=11, "WHITE BALANCE"=12, "PHOTON IMAGING MODE"=13, "HIGH DYNAMIC RANGE MODE"=14, "TRIGGER SOURCE"=15, "TRIGGER ACTIVE"=16, "TRIGGER MODE"=17, "TRIGGER POLARITY"=18, "TRIGGER GLOBAL EXPOSURE"=19, "FIRST TRIGGER BEHAVIOR"=20, "TRIGGER TIMES"=21, "OUTPUT TRIGGER POLARITY"=22, "OUTPUT TRIGGER DELAY"=23, "OUTPUT TRIGGER PERIOD"=24, "TEMPERATURE"=25, "TEMPERATURE TARGET"=26, "SENSOR COOLER FAN"=27, "MECHANICAL SHUTTER"=28, "BACK FOCUS POSITION"=29, "FRAMEBUNDLE MODE"=30, "FRAMEBUNDLE NUMBER"=31, "LINEBUNDLE HEIGHT"=32, "TRIGGER CONNECTOR"=33, "IMAGE PIXEL TYPE"=34] ("Parameter")
                          w278 = 1 items=["Snap", "Sequence"] ("Capture mode")
                          w281 = 3 items=["Edge"=1, "Level"=2, "Syncreadout"=3] ("Trigger Source")
                          w282 = 16 items=["BINNING"=1, "BITS PER CHANNEL"=2, "ACTIVE VIEW INDEX"=3, "CCD MODE"=4, "SENSOR MODE"=5, "READOUT MODE"=6, "EXPOSURE TIME"=7, "CONTRAST GAIN"=8, "CONTRAST OFFSET"=9, "LIGHT MODE"=10, "SENSITIVITY"=11, "WHITE BALANCE"=12, "PHOTON IMAGING MODE"=13, "HIGH DYNAMIC RANGE MODE"=14, "TRIGGER SOURCE"=15, "TRIGGER ACTIVE"=16, "TRIGGER MODE"=17, "TRIGGER POLARITY"=18, "TRIGGER GLOBAL EXPOSURE"=19, "FIRST TRIGGER BEHAVIOR"=20, "TRIGGER TIMES"=21, "OUTPUT TRIGGER POLARITY"=22, "OUTPUT TRIGGER DELAY"=23, "OUTPUT TRIGGER PERIOD"=24, "TEMPERATURE"=25, "TEMPERATURE TARGET"=26, "SENSOR COOLER FAN"=27, "MECHANICAL SHUTTER"=28, "BACK FOCUS POSITION"=29, "FRAMEBUNDLE MODE"=30, "FRAMEBUNDLE NUMBER"=31, "LINEBUNDLE HEIGHT"=32, "TRIGGER CONNECTOR"=33, "IMAGE PIXEL TYPE"=34] ("Parameter")
                          w284 = 2 items=["Internal"=1, "External"=2, "Software"=3] ("Trigger Source")
                          w283 = 15 items=["BINNING"=1, "BITS PER CHANNEL"=2, "ACTIVE VIEW INDEX"=3, "CCD MODE"=4, "SENSOR MODE"=5, "READOUT MODE"=6, "EXPOSURE TIME"=7, "CONTRAST GAIN"=8, "CONTRAST OFFSET"=9, "LIGHT MODE"=10, "SENSITIVITY"=11, "WHITE BALANCE"=12, "PHOTON IMAGING MODE"=13, "HIGH DYNAMIC RANGE MODE"=14, "TRIGGER SOURCE"=15, "TRIGGER ACTIVE"=16, "TRIGGER MODE"=17, "TRIGGER POLARITY"=18, "TRIGGER GLOBAL EXPOSURE"=19, "FIRST TRIGGER BEHAVIOR"=20, "TRIGGER TIMES"=21, "OUTPUT TRIGGER POLARITY"=22, "OUTPUT TRIGGER DELAY"=23, "OUTPUT TRIGGER PERIOD"=24, "TEMPERATURE"=25, "TEMPERATURE TARGET"=26, "SENSOR COOLER FAN"=27, "MECHANICAL SHUTTER"=28, "BACK FOCUS POSITION"=29, "FRAMEBUNDLE MODE"=30, "FRAMEBUNDLE NUMBER"=31, "LINEBUNDLE HEIGHT"=32, "TRIGGER CONNECTOR"=33, "IMAGE PIXEL TYPE"=34] ("Parameter")
                          # "External Trigger Mode"
                          n137 = call <userlib>:"tm_stopcapture.vi"("error in (no error)"=w240, "Handle in"=w239) -> ("error out"=w243:errorcluster, "Handle out"=w244:u32)  [unwired: 8 in]
                          n138 = flat-sequence {
                            tunnel: [w331] -> w260
                            frame #0 {
                              n139 = local read "File Name"() -> (w323:string)
                              n140 = Get Date/Time In Seconds() -> (seconds since 1Jan1904=w325:timestamp)
                              n141 = Format Date/Time String(time format string (%c)="_at%H%M%S", seconds (now)=w325) -> (date/time string=w324:string)  [unwired: 1 in]
                              n142 = local write "Status"("Acquiring movie" ("Status")) -> ()
                              n143 = local read "base path"() -> (w329:path)
                              n144 = Concatenate Strings(w323, w324, ".dcimg" ("string")) -> (w330:string)
                              n145 = Build Path(base path=w329, name or relative path=w330) -> (appended path=w331:path)
                            }
                          }
                          n146 = call <userlib>:"tm_unpreparecapture.vi"("error in (no error)"=w243, "Handle in"=w244) -> ("error out"=w241:errorcluster, "Handle out"=w242:u32)  [unwired: 8 in]
                          n147 = call <userlib>:"tm_setparameter.vi"("error in (no error)"=w241, "Value in"=w284, "Parameter"=w283, "Handle in"=w242) -> ("error out"=w279:errorcluster, "Handle out"=w280:u32)  [unwired: 6 in]
                          n148 = call <userlib>:"tm_setparameter.vi"("error in (no error)"=w279, "Value in"=w281, "Parameter"=w282, "Handle in"=w280) -> ("error out"=w276:errorcluster, "Handle out"=w277:u32)  [unwired: 6 in]
                          n149 = local read "# frames"() -> (w273:u32)
                          n150 = call <userlib>:"tm_preparecapture.vi"("error in (no error)"=w276, "Capture mode"=w278, "Handle in"=w277) -> ("error out"=w275:errorcluster, "Handle out"=w274:u32)  [unwired: 5 in, 2 out]
                          n151 = local read "# frames"() -> (w267:u32)
                          n152 = call <userlib>:"tm_startrecorder.vi"("error in (no error)"=w275, "frames"=w273, "File"=w260, "Handle in"=w274) -> ("error out"=w272:errorcluster, "Handle out"=w271:u32)  [unwired: 6 in]
                          n153 = Tick Count (ms)() -> (millisecond timer value=w270:u32)
                          n154 = call <userlib>:"tm_startcapture_b.vi"("error in (no error)"=w272, "Handle in"=w271) -> ("error out"=w269:errorcluster, "Handle out"=w268:u32)  [unwired: 8 in]
                          n155 = local read "Enter Live Mode"() -> (w257:bool)
                          n156 = case shown="No Error" w269 {
                            selector: w269 -> [w307 w322]
                            tunnel: [w305 w321] -> w265
                            tunnel: [w306 w322] -> w266
                            tunnel: w268 -> [w304 w321]
                            tunnel: w270 -> [w303 _]
                            tunnel: w267 -> [w302 _]
                            frame No Error {
                              n157 = while {
                                tunnel: w307 -> [w319]
                                tunnel: [w318] -> w306
                                tunnel: [w320] -> w305
                                tunnel: w304 -> [w312]
                                tunnel: w303 -> [w311]
                                tunnel: w302 -> [w309]
                                stop <- w317 stop-if-true
                                n158 = Tick Count (ms)() -> (millisecond timer value=w314:u32)
                                n159 = Subtract(x=w314, y=w311) -> (x-y=w313:u32)
                                n160 = call <userlib>:"tm_getrecorderstatus.vi"("error in (no error)"=w319, "Handle"=w312) -> ("error out"=w318:errorcluster, "Count"=w308:i32, "Handle"=w320:u32)  [unwired: 6 in, 1 out]
                                n161 = Divide(x=w313, y=1000.0) -> (x/y=w310:dbl)
                                n162 = local write "Frames Recorded"(w308) -> ()
                                n163 = Greater Or Equal?(x=w308, y=w309) -> (x >= y?=w317:bool)
                                n164 = local write "Elapsed time (sec)"(w310) -> ()
                                n165 = Wait (ms)(milliseconds to wait=u32 100) -> ()  [unwired: 1 out]
                              }
                            }
                            frame Error {
                            }
                          }
                          n166 = call <userlib>:"tm_stoprecorder.vi"("error in (no error)"=w266, "Handle in"=w265) -> ("error out"=w264:errorcluster, "Handle out"=w263:u32)  [unwired: 8 in]
                          n167 = local read "Exposure (msec)"() -> (w248:T4)
                          n168 = local read "Bin (n x n)"() -> (w246:u16)
                          n169 = local read "# frames"() -> (w247:u32)
                          n170 = call <userlib>:"tm_stopcapture.vi"("error in (no error)"=w264, "Handle in"=w263) -> ("error out"=w262:errorcluster, "Handle out"=w261:u32)  [unwired: 8 in]
                          n171 = local read "ROI"() -> (w245:T2)
                          n172 = call <userlib>:"tm_unpreparecapture.vi"("error in (no error)"=w262, "Handle in"=w261) -> ("error out"=w234:errorcluster, "Handle out"=w235:u32)  [unwired: 8 in]
                          n173 = call <userlib>:"tm_setparameter.vi"("error in (no error)"=w234, "Value in"=w237, "Parameter"=w238, "Handle in"=w235) -> ("error out"=w236:errorcluster)  [unwired: 6 in, 1 out]
                          n174 = call "subSaveAsBin_NW348.vi"("Delete .dcimg?"=TRUE, "Save Text file?"=TRUE, "Error in"=w236, ".dcimg file name"=w260) -> ("Error out"=w251:errorcluster, "text path"=w249:path)  [unwired: 6 in]
                          n175 = case shown="True" w257 {
                            tunnel: [w291 w298] -> w252
                            tunnel: [u32 0 ("Handle out") w297] -> w255
                            tunnel: [T6 {"width"=0, "height"=0, "datatype"=0} ("Buffer") w296] -> w256
                            tunnel: w251 -> [w291 w295]
                            frame False {
                            }
                            frame True {
                              w299 = 1 items=["Snap", "Sequence"] ("Capture mode")
                              n176 = call <userlib>:"tm_preparecapture.vi"("error in (no error)"=w295, "Capture mode"=w299, "Handle in"=u32 0) -> ("error out"=w301:errorcluster, "Buffer"=w296:T6, "Handle out"=w300:u32)  [unwired: 5 in, 1 out]
                              n177 = call <userlib>:"tm_startcapture_b.vi"("error in (no error)"=w301, "Handle in"=w300) -> ("error out"=w298:errorcluster, "Handle out"=w297:u32)  [unwired: 8 in]
                            }
                          }
                          n178 = stacked-sequence {
                            tunnel: [w290] -> w254
                            tunnel: w255 -> [w290]
                            tunnel: w252 -> [w289]
                            tunnel: [w289] -> w250
                            tunnel: w256 -> [w286]
                            tunnel: [w286] -> w253
                            frame #0 {
                              n179 = local write "Acquire movie"(FALSE ("Acquire movie")) -> ()
                              n180 = local write "Status"("Ready" ("Status")) -> ()
                              n181 = local write "Trigger"(TRUE ("Trigger")) -> ()
                            }
                          }
                          n182 = call "subSaveExperimentParams.vi"("Exposure"=w248, "Path"=w249, "ROI"=w245, "Binning"=w246, "# of Frames"=w247) -> ()  [unwired: 5 in]
                        }
                        frame True {
                          w361 = 1 items=["Snap", "Sequence"] ("Capture mode")
                          # "Internal Trigger Mode"
                          n183 = flat-sequence {
                            tunnel: [w422] -> w346
                            frame #0 {
                              n184 = local read "File Name"() -> (w414:string)
                              n185 = Get Date/Time In Seconds() -> (seconds since 1Jan1904=w416:timestamp)
                              n186 = Format Date/Time String(time format string (%c)="_at%H%M%S", seconds (now)=w416) -> (date/time string=w415:string)  [unwired: 1 in]
                              n187 = local write "Status"("Acquiring movie" ("Status")) -> ()
                              n188 = local read "base path"() -> (w420:path)
                              n189 = Concatenate Strings(w414, w415, ".dcimg" ("string")) -> (w421:string)
                              n190 = Build Path(base path=w420, name or relative path=w421) -> (appended path=w422:path)
                            }
                          }
                          n191 = local read "Enter Live Mode"() -> (w366:bool)
                          n192 = case shown="True" w366 {
                            tunnel: [w407 w411] -> w359
                            tunnel: w368 -> [w407 w410]
                            tunnel: w367 -> [w406 w409]
                            tunnel: [w406 w408] -> w360
                            frame False {
                            }
                            frame True {
                              n193 = call <userlib>:"tm_stopcapture.vi"("error in (no error)"=w410, "Handle in"=w409) -> ("error out"=w412:errorcluster, "Handle out"=w413:u32)  [unwired: 8 in]
                              n194 = call <userlib>:"tm_unpreparecapture.vi"("error in (no error)"=w412, "Handle in"=w413) -> ("error out"=w411:errorcluster, "Handle out"=w408:u32)  [unwired: 8 in]
                            }
                          }
                          n195 = call <userlib>:"tm_preparecapture.vi"("error in (no error)"=w359, "Capture mode"=w361, "Handle in"=w360) -> ("error out"=w362:errorcluster, "Handle out"=w363:u32)  [unwired: 5 in, 2 out]
                          n196 = local read "# frames"() -> (w339:u32)
                          n197 = call <userlib>:"tm_startrecorder.vi"("error in (no error)"=w362, "frames"=w339, "File"=w346, "Handle in"=w363) -> ("error out"=w364:errorcluster, "Handle out"=w365:u32)  [unwired: 6 in]
                          n198 = call <userlib>:"tm_startcapture_b.vi"("error in (no error)"=w364, "Handle in"=w365) -> ("error out"=w358:errorcluster, "Handle out"=w357:u32)  [unwired: 8 in]
                          n199 = Tick Count (ms)() -> (millisecond timer value=w347:u32)
                          n200 = case shown="No Error" w358 {
                            selector: w358 -> [w390 w405]
                            tunnel: [w388 w404] -> w351
                            tunnel: [w389 w405] -> w352
                            tunnel: w357 -> [w387 w404]
                            tunnel: w347 -> [w386 _]
                            tunnel: w339 -> [w385 _]
                            frame No Error {
                              n201 = while {
                                tunnel: w390 -> [w402]
                                tunnel: [w401] -> w389
                                tunnel: [w403] -> w388
                                tunnel: w387 -> [w395]
                                tunnel: w386 -> [w392]
                                tunnel: w385 -> [w391]
                                stop <- w400 stop-if-true
                                n202 = Tick Count (ms)() -> (millisecond timer value=w397:u32)
                                n203 = Subtract(x=w397, y=w392) -> (x-y=w396:u32)
                                n204 = call <userlib>:"tm_getrecorderstatus.vi"("error in (no error)"=w402, "Handle"=w395) -> ("error out"=w401:errorcluster, "Count"=w394:i32, "Handle"=w403:u32)  [unwired: 6 in, 1 out]
                                "Frames Recorded" <- w394
                                n205 = Divide(x=w396, y=1000.0) -> (x/y=→"Elapsed time (sec)":dbl)
                                n206 = Greater Or Equal?(x=w394, y=w391) -> (x >= y?=w400:bool)
                                n207 = Wait (ms)(milliseconds to wait=u32 100) -> ()  [unwired: 1 out]
                              }
                            }
                            frame Error {
                            }
                          }
                          n208 = local read "Enter Live Mode"() -> (w344:bool)
                          n209 = call <userlib>:"tm_stoprecorder.vi"("error in (no error)"=w352, "Handle in"=w351) -> ("error out"=w356:errorcluster, "Handle out"=w355:u32)  [unwired: 8 in]
                          n210 = local read "Exposure (msec)"() -> (w336:T4)
                          n211 = call <userlib>:"tm_stopcapture.vi"("error in (no error)"=w356, "Handle in"=w355) -> ("error out"=w353:errorcluster, "Handle out"=w354:u32)  [unwired: 8 in]
                          n212 = local read "Bin (n x n)"() -> (w334:u16)
                          n213 = local read "# frames"() -> (w335:u32)
                          n214 = local read "ROI"() -> (w333:T2)
                          n215 = call <userlib>:"tm_unpreparecapture.vi"("error in (no error)"=w353, "Handle in"=w354) -> ("error out"=w350:errorcluster)  [unwired: 8 in, 1 out]
                          n216 = call "subSaveAsBin_NW348.vi"("Delete .dcimg?"=TRUE, "Save Text file?"=TRUE, "Error in"=w350, ".dcimg file name"=w346) -> ("Error out"=w345:errorcluster, "text path"=w332:path)  [unwired: 6 in]
                          n217 = case shown="True" w344 {
                            tunnel: [w374 w381] -> w342
                            tunnel: [u32 0 ("Handle out") w380] -> w343
                            tunnel: [T6 {"width"=0, "height"=0, "datatype"=0} ("Buffer") w379] -> w338
                            tunnel: w345 -> [w374 w378]
                            frame False {
                            }
                            frame True {
                              w382 = 1 items=["Snap", "Sequence"] ("Capture mode")
                              n218 = call <userlib>:"tm_preparecapture.vi"("error in (no error)"=w378, "Capture mode"=w382, "Handle in"=u32 0) -> ("error out"=w384:errorcluster, "Buffer"=w379:T6, "Handle out"=w383:u32)  [unwired: 5 in, 1 out]
                              n219 = call <userlib>:"tm_startcapture_b.vi"("error in (no error)"=w384, "Handle in"=w383) -> ("error out"=w381:errorcluster, "Handle out"=w380:u32)  [unwired: 8 in]
                            }
                          }
                          n220 = stacked-sequence {
                            tunnel: [w373] -> w341
                            tunnel: w343 -> [w373]
                            tunnel: w342 -> [w372]
                            tunnel: [w372] -> w340
                            tunnel: w338 -> [w369]
                            tunnel: [w369] -> w337
                            frame #0 {
                              n221 = local write "Acquire movie"(FALSE ("Acquire movie")) -> ()
                              n222 = local write "Status"("Ready" ("Status")) -> ()
                            }
                          }
                          n223 = call "subSaveExperimentParams.vi"("Exposure"=w336, "Path"=w332, "ROI"=w333, "Binning"=w334, "# of Frames"=w335) -> ()  [unwired: 5 in]
                        }
                      }
                    }
                    event Value Change {
                      w430 = 7 items=["BINNING"=1, "BITS PER CHANNEL"=2, "ACTIVE VIEW INDEX"=3, "CCD MODE"=4, "SENSOR MODE"=5, "READOUT MODE"=6, "EXPOSURE TIME"=7, "CONTRAST GAIN"=8, "CONTRAST OFFSET"=9, "LIGHT MODE"=10, "SENSITIVITY"=11, "WHITE BALANCE"=12, "PHOTON IMAGING MODE"=13, "HIGH DYNAMIC RANGE MODE"=14, "TRIGGER SOURCE"=15, "TRIGGER ACTIVE"=16, "TRIGGER MODE"=17, "TRIGGER POLARITY"=18, "TRIGGER GLOBAL EXPOSURE"=19, "FIRST TRIGGER BEHAVIOR"=20, "TRIGGER TIMES"=21, "OUTPUT TRIGGER POLARITY"=22, "OUTPUT TRIGGER DELAY"=23, "OUTPUT TRIGGER PERIOD"=24, "TEMPERATURE"=25, "TEMPERATURE TARGET"=26, "SENSOR COOLER FAN"=27, "MECHANICAL SHUTTER"=28, "BACK FOCUS POSITION"=29, "FRAMEBUNDLE MODE"=30, "FRAMEBUNDLE NUMBER"=31, "LINEBUNDLE HEIGHT"=32, "TRIGGER CONNECTOR"=33, "IMAGE PIXEL TYPE"=34] ("Parameter")
                      n224 = event-data() -> ()  [unwired: 1 in, 5 out]
                      n225 = local read "Exposure (msec)"() -> (w426:T4)
                      n226 = Divide(x=w426, y=1000.0) -> (x/y=w425:T4)
                      n227 = call <userlib>:"tm_setparameter.vi"("error in (no error)"=w427, "Value in"=w425, "Parameter"=w430, "Handle in"=w431) -> ("error out"=w428:errorcluster, "Handle out"=w429:u32)  [unwired: 6 in]
                    }
                    event "Bin (n x n)": Value Change {
                      w447 = 1 items=["Snap", "Sequence"] ("Capture mode")
                      n228 = event-data() -> ("OldVal"=w435:u16, "NewVal"=w434:u16)  [unwired: 1 in]
                      n229 = call <userlib>:"tm_stopcapture.vi"("error in (no error)"=w472, "Handle in"=w473) -> ("error out"=w470:errorcluster, "Handle out"=w471:u32)  [unwired: 8 in]
                      n230 = call <userlib>:"tm_unpreparecapture.vi"("error in (no error)"=w470, "Handle in"=w471) -> ("error out"=w468:errorcluster, "Handle out"=w469:u32)  [unwired: 8 in]
                      n231 = property on="Image" class="IntGraph (strict)"() -> ("XScale.Minimum"=w465:dbl, "YScale.Minimum"=w466:dbl, "XScale.Maximum"=w464:dbl, "YScale.Maximum"=w463:dbl)  [unwired: 2 in, 2 out]
                      n232 = property on="Image" class="IntGraph (strict)"("Active Cursor"=u32 1) -> ("Cursor.Cursor Position"=w458:T13)  [unwired: 2 in, 2 out]
                      n233 = property on="Image" class="IntGraph (strict)"("Active Cursor"=u32 0) -> ("Cursor.Cursor Position"=w459:T13)  [unwired: 2 in, 2 out]
                      n234 = local read "x pixels"() -> (w438:i32)
                      n235 = Bundle("XScale.Minimum"=w465, "YScale.Minimum"=w466, "XScale.Maximum"=w464, "YScale.Maximum"=w463) -> (w462:T14)  [unwired: 1 in]
                      n236 = local read "ROI"() -> (w467:T2)
                      n237 = Bundle("Cursor.Cursor Position"=w459, "Cursor.Cursor Position"=w458) -> (w457:T15)  [unwired: 1 in]
                      n238 = call "subUpdateCameraBin_NW348.vi"("Bin (n x n)"=w434, "Previous bin"=w435, "Cursor in"=w457, "Error in (no error)"=w468, "Graph scale in"=w462, "ROI in"=w467, "Handle in"=w469) -> ("Error out"=w442:errorcluster, "Graph scale out"=w432:T14, "ROI out"=w433:T2, "Handle out"=w443:u32, "Cursor out"=w454:T16)
                      n239 = Divide(x=w438, y="Bin (n x n)") -> (x/y=w436:dbl)
                      n240 = local write "ROI"(w433) -> ()
                      n241 = call "subUpdateLocIndicator_NW348.vi"("ROI"=w433, "pixel range"=w436) -> ("Location indicator"=w437:u16[][])  [unwired: 8 in, 1 out]
                      n242 = Unbundle By Name(w432) -> ("XScale.Minimum"=w451:dbl, "YScale.Minimum"=w450:dbl, "XScale.Maximum"=w449:dbl, "YScale.Maximum"=w448:dbl)
                      n243 = Unbundle(w454) -> ("Cursor1.Position"=w453:T13, "Cursor2.Position"=w452:T13)
                      n244 = local write "Location indicator"(w437) -> ()
                      n245 = property on="Image" class="IntGraph (strict)"("XScale.Minimum"=w451, "YScale.Minimum"=w450, "XScale.Maximum"=w449, "YScale.Maximum"=w448) -> ()  [unwired: 2 in, 2 out]
                      n246 = property on="Image" class="IntGraph (strict)"("Active Cursor"=u32 0, "Cursor.Cursor Position"=w453) -> ()  [unwired: 2 in, 2 out]
                      n247 = property on="Image" class="IntGraph (strict)"("Active Cursor"=u32 1, "Cursor.Cursor Position"=w452) -> ()  [unwired: 2 in, 2 out]
                      n248 = call <userlib>:"tm_preparecapture.vi"("error in (no error)"=w442, "Capture mode"=w447, "Handle in"=w443) -> ("error out"=w445:errorcluster, "Buffer"=w444:T6, "Handle out"=w446:u32)  [unwired: 5 in, 1 out]
                      n249 = call <userlib>:"tm_startcapture_b.vi"("error in (no error)"=w445, "Handle in"=w446) -> ("error out"=w440:errorcluster, "Handle out"=w441:u32)  [unwired: 8 in]
                    }
                    event "Update ROI", "ROI": Value Change {
                      w490 = 1 items=["Snap", "Sequence"] ("Capture mode")
                      n250 = event-data() -> ()  [unwired: 1 in, 1 out]
                      n251 = call <userlib>:"tm_stopcapture.vi"("error in (no error)"=w479, "Handle in"=w478) -> ("error out"=w477:errorcluster, "Handle out"=w476:u32)  [unwired: 8 in]
                      n252 = call <userlib>:"tm_unpreparecapture.vi"("error in (no error)"=w477, "Handle in"=w476) -> ("error out"=w475:errorcluster, "Handle out"=w474:u32)  [unwired: 8 in]
                      n253 = flat-sequence {
                        tunnel: [w503] -> w497
                        tunnel: [w502] -> w496
                        tunnel: [w501] -> w495
                        tunnel: w474 -> [w501]
                        tunnel: w475 -> [w500]
                        tunnel: [w500] -> w493
                        tunnel: ["ROI selection"] -> w480
                        tunnel: w497 -> [_]
                        tunnel: w496 -> [w514]
                        tunnel: w495 -> [w513]
                        tunnel: [w512] -> w494
                        tunnel: w493 -> [w511]
                        tunnel: [w510] -> w492
                        tunnel: [w509] -> w491
                        tunnel: [w508] -> w482
                        tunnel: [w507] -> w481
                        tunnel: w480 -> [w506]
                        tunnel: w494 -> [w601]
                        tunnel: w492 -> [w602]
                        tunnel: w491 -> [w600]
                        tunnel: [w596] -> w484
                        tunnel: [w595] -> w483
                        tunnel: w482 -> [w577]
                        tunnel: w481 -> [w576]
                        frame #0 {
                          n254 = local read "ROI"() -> (→"Previous ROI":T2)
                          n255 = local read "Bin (n x n)"() -> (w503:u16)
                          "Previous Bin" <- w503
                          n256 = local write "Update ROI"(FALSE ("Update ROI")) -> ()
                          n257 = property on="Previous ROI" class="Clust (strict)"("DisabledEnum"=T5."Enabled" ("Disabled")) -> ()  [unwired: 2 in, 2 out]
                          n258 = local read "Draw ROI"() -> (w502:bool)
                        }
                        frame #1 {
                          n259 = case shown="False" w514 {
                            tunnel: [w515 w565] -> w512
                            tunnel: w513 -> [w516 w565]
                            tunnel: w511 -> [w517 w564]
                            tunnel: [w517 w564] -> w510
                            tunnel: [w520 w563] -> w508
                            tunnel: [w519 w562] -> w509
                            tunnel: w506 -> [w518 _]
                            frame False {
                              n260 = case shown="3" w518 {
                                tunnel: [w523 w532 w549 w554] -> w520
                                tunnel: [w522 w531 w538 w560] -> w519
                                tunnel: w516 -> [w521 w528 w548 w559]
                                tunnel: [w521 w528 w548 w559] -> w515
                                frame 0, Default {
                                w523 = u16 4 items=["1x1"=1, "2x2"=2, "4x4"=4] ("Bin (n x n)")
                                w526 = u32 0 ("Active Cursor")
                                n261 = local read "x pixels"() -> (w525:i32)
                                n262 = local read "Previous Bin"() -> (w524:u16)
                                n263 = Divide(x=w525, y=w524) -> (x/y=w527:dbl)
                                n264 = local write "Bin (n x n)"(w523) -> ()
                                n265 = Bundle("Active Cursor"=w526, "Active Cursor"=w526, w527, w527) -> (w522:T17)  [unwired: 1 in]
                                }
                                frame 1 {
                                w532 = u16 2 items=["1x1"=1, "2x2"=2, "4x4"=4] ("Bin (n x n)")
                                # "Central quadrant"
                                n266 = local read "x pixels"() -> (w529:i32)
                                n267 = local read "Previous Bin"() -> (w530:u16)
                                n268 = Divide(x=w529, y=w530) -> (x/y=w533:dbl)
                                n269 = local write "Bin (n x n)"(w532) -> ()
                                n270 = Multiply(x=0.25, y=w533) -> (x*y=w536:dbl)
                                n271 = Multiply(x=w533, y=0.5) -> (x*y=w534:dbl)
                                n272 = Bundle(w536, w536, w534, w534) -> (w531:cluster{dbl, dbl, dbl, dbl})  [unwired: 1 in]
                                }
                                frame 2 {
                                w549 = u16 1 items=["1x1"=1, "2x2"=2, "4x4"=4] ("Bin (n x n)")
                                # "Red Laser ROI"
                                # "ywidth"
                                # "xwidth"
                                # "yoffset"
                                # "xoffset"
                                n273 = local read "Previous Bin"() -> (w539:u16)
                                n274 = Divide(x=512.0, y=w539) -> (x/y=w543:dbl)
                                n275 = Divide(x=844.0, y=w539) -> (x/y=w544:dbl)
                                n276 = Divide(x=1024.0, y=w539) -> (x/y=w546:dbl)
                                n277 = Divide(x=360.0, y=w539) -> (x/y=w547:dbl)
                                n278 = local write "Bin (n x n)"(w549) -> ()
                                n279 = Bundle(w543, w544, w546, w547) -> (w538:cluster{dbl, dbl, dbl, dbl})  [unwired: 1 in]
                                }
                                frame 3 {
                                n280 = local read "Previous Bin"() -> (w554:u16)
                                n281 = local read "ROI"() -> (w561:T2)
                                n282 = Unbundle By Name(w561) -> ("x offset"=w558:i32, "y offset"=w555:i32, "x width"=w556:i32, "y width"=w557:i32)
                                n283 = local write "Bin (n x n)"(w554) -> ()
                                n284 = To Double Precision Float(number=w558) -> (double precision float=w553:dbl)
                                n285 = To Double Precision Float(number=w555) -> (double precision float=w552:dbl)
                                n286 = To Double Precision Float(number=w556) -> (double precision float=w551:dbl)
                                n287 = To Double Precision Float(number=w557) -> (double precision float=w550:dbl)
                                n288 = Bundle(w553, w552, w551, w550) -> (w560:cluster{dbl, dbl, dbl, dbl})  [unwired: 1 in]
                                }
                              }
                            }
                            frame True {
                              w563 = u16 1 items=["1x1"=1, "2x2"=2, "4x4"=4] ("Bin (n x n)")
                              w566 = u16 2 items=["Full ROI", "Central quad", "Custom ROI"] ("ROI selection")
                              w567 = FALSE ("Define ROI")
                              n289 = local read "ROI cursor"() -> (w562:T2)
                              n290 = local write "ROI selection"(w566) -> ()
                              n291 = local write "Draw ROI"(w567) -> ()
                              n292 = property on="Image" class="IntGraph (strict)"("Active Cursor"=u32 0, "Cursor.Visible"=w567) -> ()  [unwired: 2 in, 2 out]
                              n293 = property on="Image" class="IntGraph (strict)"("Active Cursor"=u32 1, "Cursor.Visible"=w567) -> ()  [unwired: 2 in, 2 out]
                              n294 = local write "Bin (n x n)"(w563) -> ()
                            }
                          }
                          n295 = local read "Previous Bin"() -> (w507:u16)
                        }
                        frame #2 {
                          n296 = local read "x pixels"() -> (w585:i32)
                          n297 = local read "Bin (n x n)"() -> (w586:u16)
                          n298 = call "subUpdateCameraBin_NW348.vi"("Bin (n x n)"=w577, "Previous bin"=w576, "Error in (no error)"=w602, "ROI in"=w600, "Handle in"=w601) -> ("Error out"=w598:errorcluster, "ROI out"=w571:T2, "Handle out"=w599:u32)  [unwired: 2 in, 2 out]
                          n299 = local read "Bin (n x n)"() -> (w574:u16)
                          n300 = local read "x pixels"() -> (w573:i32)
                          n301 = local read "Bin (n x n)"() -> (w570:u16)
                          n302 = call "subImageROI2CameraROI_NW348.vi"("image ROI"=w571) -> ("camera ROI"=w597:T2)
                          n303 = Unbundle By Name(w571) -> ("x offset"=w589:i32, "y offset"=w590:i32, "x width"=w592:i32, "y width"=w591:i32)
                          n304 = local write "ROI"(w571) -> ()
                          n305 = Divide(x=w585, y=w586) -> (x/y=w584:dbl)
                          n306 = call "subUpdateLocIndicator_NW348.vi"("ROI"=w571, "pixel range"=w584) -> ("Graph scale"=w583:T9, "Location indicator"=w578:u16[][])  [unwired: 8 in]
                          n307 = Divide(x=w573, y=w574) -> (x/y=w572:dbl)
                          n308 = Unbundle By Name(w583) -> ("X min"=w582:dbl, "Y min"=w581:dbl, "X max"=w580:dbl, "Y max"=w579:dbl)
                          n309 = call <userlib>:"tm_setarea.vi"("error in (no error)"=w598, "Sub Region"=w597, "Handle in"=w599) -> ("error out"=w595:errorcluster, "Handle out"=w596:u32)  [unwired: 7 in]
                          n310 = Add(x=w592, y=w589) -> (x+y=w588:i32)
                          n311 = call "subGetMaxCameraRate_cokeCan.vi"("Bin (n x n)"=w570, "ROI"=w571, "Binned pixels"=w572) -> ("max frame rate (Hz)"=→"max frame rate (Hz)":dbl)  [unwired: 8 in]
                          n312 = Add(x=w591, y=w590) -> (x+y=w587:i32)
                          n313 = local write "Location indicator"(w578) -> ()
                          n314 = property on="Image" class="IntGraph (strict)"("XScale.Minimum"=w582, "YScale.Minimum"=w581, "XScale.Maximum"=w580, "YScale.Maximum"=w579) -> ()  [unwired: 2 in, 2 out]
                          n315 = property on="Image" class="IntGraph (strict)"("Active Cursor"=u32 0, "Cursor.Cursor X"=w589, "Cursor.Cursor Y"=w590) -> ()  [unwired: 2 in, 2 out]
                          n316 = property on="Image" class="IntGraph (strict)"("Active Cursor"=u32 1, "Cursor.Cursor X"=w588, "Cursor.Cursor Y"=w587) -> ()  [unwired: 2 in, 2 out]
                        }
                      }
                      n317 = call <userlib>:"tm_preparecapture.vi"("error in (no error)"=w483, "Capture mode"=w490, "Handle in"=w484) -> ("error out"=w489:errorcluster, "Buffer"=w485:T6, "Handle out"=w488:u32)  [unwired: 5 in, 1 out]
                      n318 = call <userlib>:"tm_startcapture_b.vi"("error in (no error)"=w489, "Handle in"=w488) -> ("error out"=w486:errorcluster, "Handle out"=w487:u32)  [unwired: 8 in]
                    }
                    event "Draw ROI": Value Change {
                      n319 = event-data() -> ()  [unwired: 1 in, 1 out]
                      n320 = case shown="True" "Draw ROI" {
                        frame False {
                          w607 = FALSE ("Cursor.Visible")
                          n321 = property on="Image" class="IntGraph (strict)"("Active Cursor"=u32 0, "Cursor.Visible"=w607) -> ()  [unwired: 2 in, 2 out]
                          n322 = property on="Image" class="IntGraph (strict)"("Active Cursor"=u32 1, "Cursor.Visible"=w607) -> ()  [unwired: 2 in, 2 out]
                        }
                        frame True {
                          w610 = TRUE ("Cursor.Visible")
                          n323 = property on="Image" class="IntGraph (strict)"() -> ("XScale.Minimum"=w612:dbl, "YScale.Minimum"=w611:dbl, "XScale.Maximum"=w614:dbl, "YScale.Maximum"=w613:dbl)  [unwired: 2 in, 2 out]
                          n324 = property on="Image" class="IntGraph (strict)"("Active Cursor"=u32 0, "Cursor.Visible"=w610, "Cursor.Cursor X"=w612, "Cursor.Cursor Y"=w611) -> ()  [unwired: 2 in, 2 out]
                          n325 = property on="Image" class="IntGraph (strict)"("Active Cursor"=u32 1, "Cursor.Visible"=w610, "Cursor.Cursor X"=w614, "Cursor.Cursor Y"=w613) -> ()  [unwired: 2 in, 2 out]
                        }
                      }
                    }
                    event "Previous ROI 2": Value Change {
                      w617 = FALSE ("Define ROI")
                      w631 = 1 items=["Snap", "Sequence"] ("Capture mode")
                      w646 = 1 items=["BINNING"=1, "BITS PER CHANNEL"=2, "ACTIVE VIEW INDEX"=3, "CCD MODE"=4, "SENSOR MODE"=5, "READOUT MODE"=6, "EXPOSURE TIME"=7, "CONTRAST GAIN"=8, "CONTRAST OFFSET"=9, "LIGHT MODE"=10, "SENSITIVITY"=11, "WHITE BALANCE"=12, "PHOTON IMAGING MODE"=13, "HIGH DYNAMIC RANGE MODE"=14, "TRIGGER SOURCE"=15, "TRIGGER ACTIVE"=16, "TRIGGER MODE"=17, "TRIGGER POLARITY"=18, "TRIGGER GLOBAL EXPOSURE"=19, "FIRST TRIGGER BEHAVIOR"=20, "TRIGGER TIMES"=21, "OUTPUT TRIGGER POLARITY"=22, "OUTPUT TRIGGER DELAY"=23, "OUTPUT TRIGGER PERIOD"=24, "TEMPERATURE"=25, "TEMPERATURE TARGET"=26, "SENSOR COOLER FAN"=27, "MECHANICAL SHUTTER"=28, "BACK FOCUS POSITION"=29, "FRAMEBUNDLE MODE"=30, "FRAMEBUNDLE NUMBER"=31, "LINEBUNDLE HEIGHT"=32, "TRIGGER CONNECTOR"=33, "IMAGE PIXEL TYPE"=34] ("Parameter")
                      w647 = u16 2 items=["Full ROI", "Central quad", "Custom ROI"] ("ROI selection")
                      n326 = event-data() -> ()  [unwired: 1 in, 1 out]
                      n327 = call <userlib>:"tm_stopcapture.vi"("error in (no error)"=w619, "Handle in"=w620) -> ("error out"=w624:errorcluster, "Handle out"=w623:u32)  [unwired: 8 in]
                      n328 = local write "Previous ROI 2"(w617) -> ()
                      n329 = local write "Draw ROI"(w617) -> ()
                      n330 = property on="Image" class="IntGraph (strict)"("Active Cursor"=u32 0, "Cursor.Visible"=w617) -> ()  [unwired: 2 in, 2 out]
                      n331 = property on="Image" class="IntGraph (strict)"("Active Cursor"=u32 1, "Cursor.Visible"=w617) -> ()  [unwired: 2 in, 2 out]
                      n332 = call <userlib>:"tm_unpreparecapture.vi"("error in (no error)"=w624, "Handle in"=w623) -> ("error out"=w621:errorcluster, "Handle out"=w622:u32)  [unwired: 8 in]
                      n333 = stacked-sequence {
                        seq-local: [w651 _ _] -> [_ _ w655]
                        seq-local: [w650 _ _] -> [_ _ w654]
                        tunnel: [_ w653 _] -> w643
                        tunnel: [_ w652 _] -> w635
                        frame #0 {
                          n334 = local read "ROI"() -> (w651:T2)
                          n335 = local read "Bin (n x n)"() -> (w650:u16)
                        }
                        frame #1 {
                          n336 = local read "Previous ROI"() -> (w652:T2)
                          n337 = local read "Previous Bin"() -> (w653:u16)
                          n338 = local write "Bin (n x n)"(w653) -> ()
                          n339 = local write "ROI"(w652) -> ()
                        }
                        frame #2 {
                          n340 = local write "Previous ROI"(w655) -> ()
                          n341 = local write "Previous Bin"(w654) -> ()
                        }
                      }
                      n342 = local write "ROI selection"(w647) -> ()
                      n343 = call <userlib>:"tm_setparameter.vi"("error in (no error)"=w621, "Value in"=w643, "Parameter"=w646, "Handle in"=w622) -> ("error out"=w633:errorcluster, "Handle out"=w632:u32)  [unwired: 6 in]
                      n344 = local read "x pixels"() -> (w644:i32)
                      n345 = Divide(x=w644, y=w643) -> (x/y=w645:dbl)
                      n346 = call "subImageROI2CameraROI_NW348.vi"("image ROI"=w635) -> ("camera ROI"=w634:T2)
                      n347 = call "subUpdateLocIndicator_NW348.vi"("ROI"=w635, "pixel range"=w645) -> ("Graph scale"=w641:T9, "Location indicator"=w642:u16[][])  [unwired: 8 in]
                      n348 = call <userlib>:"tm_setarea.vi"("error in (no error)"=w633, "Sub Region"=w634, "Handle in"=w632) -> ("error out"=w627:errorcluster, "Handle out"=w628:u32)  [unwired: 7 in]
                      n349 = Unbundle By Name(w641) -> ("X min"=w640:dbl, "Y min"=w639:dbl, "X max"=w638:dbl, "Y max"=w637:dbl)
                      n350 = local write "Location indicator"(w642) -> ()
                      n351 = call <userlib>:"tm_preparecapture.vi"("error in (no error)"=w627, "Capture mode"=w631, "Handle in"=w628) -> ("error out"=w629:errorcluster, "Buffer"=w618:T6, "Handle out"=w630:u32)  [unwired: 5 in, 1 out]
                      n352 = property on="Image" class="IntGraph (strict)"("XScale.Minimum"=w640, "YScale.Minimum"=w639, "XScale.Maximum"=w638, "YScale.Maximum"=w637) -> ()  [unwired: 2 in, 2 out]
                      n353 = Wait (ms)(milliseconds to wait=u32 200) -> ()  [unwired: 1 out]
                      n354 = call <userlib>:"tm_startcapture_b.vi"("error in (no error)"=w629, "Handle in"=w630) -> ("error out"=w625:errorcluster, "Handle out"=w626:u32)  [unwired: 8 in]
                    }
                    event "# frames": Value Change {
                      n355 = event-data() -> ()  [unwired: 1 in, 1 out]
                      n356 = local read "Exposure (msec)"() -> (w660:T4)
                      n357 = local read "# frames"() -> (w661:u32)
                      n358 = Multiply(x=w661, y=w660) -> (x*y=w659:T4)
                      n359 = Divide(x=w659, y=1000) -> (x/y=→"Total time (sec)":T4)
                    }
                    event "Snap and Save": Value Change {
                      n360 = event-data() -> ()  [unwired: 1 in, 1 out]
                      n361 = flat-sequence {
                        tunnel: [w682] -> w662
                        frame #0 {
                          n362 = local read "File Name"() -> (w683:string)
                          n363 = Get Date/Time In Seconds() -> (seconds since 1Jan1904=w685:timestamp)
                          n364 = Format Date/Time String(time format string (%c)="_at%H%M%S", seconds (now)=w685) -> (date/time string=w684:string)  [unwired: 1 in]
                          n365 = local write "Status"("Acquiring snapshot" ("Status")) -> ()
                          n366 = local read "base path"() -> (w689:path)
                          n367 = Concatenate Strings(w683, w684, ".tiff" ("string")) -> (w690:string)
                          n368 = Build Path(base path=w689, name or relative path=w690) -> (appended path=w682:path)
                        }
                      }
                      n369 = flat-sequence {
                        tunnel: w662 -> [w672]
                        frame #0 {
                          n370 = Strip Path(path=w672) -> (stripped path=w674:path, name=w677:string)
                          n371 = Search and Replace String(input string=w677, search string=".tiff", replace string=".txt" ("replace string (\"\")")) -> (result string=w673:string)  [unwired: 5 in, 3 out]
                          n372 = Build Path(base path=w674, name or relative path=w673) -> (appended path=w671:path)
                          n373 = local read "Exposure (msec)"() -> (w680:T4)
                          n374 = local read "Bin (n x n)"() -> (w679:u16)
                          n375 = local read "ROI"() -> (w678:T2)
                          n376 = call "subSaveExperimentParams.vi"("Exposure"=w680, "Path"=w671, "ROI"=w678, "Binning"=w679, "# of Frames"=1) -> ()  [unwired: 5 in]
                        }
                        frame #1 {
                          n377 = local write "Status"("Ready" ("Status")) -> ()
                        }
                      }
                      n378 = local read "Matlab Error"() -> (w664:errorcluster)
                      n379 = Path To String(path=w662) -> (string=w666:string)
                      n380 = script code="% convert data to 16-bit image\nimage = uint16(data);\n\n% open file to write or add\nt = Tiff(fileName,'a');\n\n% edit tag\ntagstruct.ImageLength = size(image, 1);\ntagstruct.ImageWidth = size(image, 2);\ntagstruct.Photometric = Tiff.Photometric.MinIsBlack;\ntagstruct.SampleFormat = Tiff.SampleFormat.IEEEFP;\ntagstruct.Compression = Tiff.Compression.None;\ntagstruct.BitsPerSample = 16;\ntagstruct.SampleFormat = Tiff.SampleFormat.UInt;\ntagstruct.SamplesPerPixel = 1;\ntagstruct.PlanarConfiguration = Tiff.PlanarConfiguration.Chunky;\ntagstruct.Software = 'MATLAB';\n\n% write file\nt.setTag(tagstruct);\nt.write(image);\nt.close();"("??"=w664, "data"=w667, "fileName"=w666) -> ("??"=w663:errorcluster)
                      n381 = local write "Matlab Error"(w663) -> ()
                    }
                    event "Define Object": Value Change {
                      n382 = event-data() -> ()  [unwired: 1 in, 1 out]
                      n383 = local read "Transformation path"() -> (w698:path)
                      n384 = local read "ROI"() -> (w703:T2)
                      n385 = local read "Bin (n x n)"() -> (w694:u16)
                      n386 = Path To String(path=w698) -> (string=w697:string)
                      n387 = Unbundle By Name(w703) -> ("x offset"=w701:i32, "y offset"=w700:i32)
                      n388 = script code="cd 'X:\\Lab\\Computer Code\\Image Processing\\Lukas_DMD_code'\n\n% clear previous roi_points cell array and roi objects\nclear roi_points; \nclear roi_objects; \nclf; \n\n% define roi points\nroi_points = clicky_stripped(data); \nnum_obj = numel(roi_points); \n\n% read in transformation matrix\ntform = dlmread(tpath); \n\n% Add xoffset and yoffset and create roi objects (in terms of 1x1 bin)\nfor i = 1:num_obj\n    roi_points{i}(:,1) = (roi_points{i}(:,1) + xoffset) * bin;\n    roi_points{i}(:,2) = (roi_points{i}(:,2) + yoffset) * bin;\n    roi_objects(i) = roi(roi_points(i), tform); \nend"("xoffset"=w701, "yoffset"=w700, "data"=w699, "tpath"=w697, "bin"=w694) -> ("??"=w693:errorcluster, "num_obj"=w692:dbl)  [unwired: 1 in]
                      n389 = local write "Matlab Error"(w693) -> ()
                      n390 = local write "# of Objects"(w692) -> ()
                      n391 = local write "Movie Complete"(FALSE ("Movie Complete")) -> ()
                    }
                    event "Make Movie": Value Change {
                      n392 = event-data() -> ()  [unwired: 1 in, 1 out]
                      n393 = flat-sequence {
                        frame #0 {
                          n394 = local read "Clicky Movie Path"() -> (w707:path)
                          n395 = Path To String(path=w707) -> (string=w706:string)
                          n396 = script code="% create fov object\nfov1 = fov(1080, 1920, 1); \n\n% Add the roi objects to the field of view\nfor i = 1:numel(roi_objects)\nfov1.add_obj(roi_objects(i), 1); \nend\n\n% Write that movie to binary\nmovie_to_bin(fov1.data, mpath);"("mpath"=w706) -> ("??"=w705:errorcluster)  [unwired: 1 in]
                          n397 = local write "Matlab Error"(w705) -> ()
                        }
                        frame #1 {
                          n398 = local write "Movie Complete"(TRUE ("Movie Complete")) -> ()
                        }
                      }
                    }
                    event "Play Movie": Value Change {
                      n399 = event-data() -> ()  [unwired: 1 in, 1 out]
                      n400 = local read "Select Mov"() -> (w709:bool)
                      n401 = case shown="True" w709 {
                        tunnel: [w713 w714] -> w710
                        frame False {
                          n402 = local read "User Movie Path"() -> (w713:path)
                        }
                        frame True {
                          n403 = local read "Clicky Movie Path"() -> (w714:path)
                        }
                      }
                      n404 = local read "Play Movie"() -> (w711:bool)
                      n405 = case shown="False" w711 {
                        tunnel: w710 -> [_ w732]
                        frame False {
                          n406 = flat-sequence {
                            frame #0 {
                              n407 = local read "DeviceID"() -> (w718:u32)
                              n408 = local read "SequID"() -> (w717:u32)
                              n409 = property on="Image Registration" class="Bool (strict)"("DisabledEnum"=T5."Enabled" ("Disabled")) -> ()  [unwired: 2 in, 2 out]
                              n410 = call "sub_remove_DMD_mov.vi"("SequenceId"=w717, "DeviceId"=w718) -> ("SeqFreeErr"=w719:i32, "DevFreeErr"=w720:i32)
                              n411 = property on="All On" class="Bool (strict)"("DisabledEnum"=T5."Enabled" ("Disabled")) -> ()  [unwired: 2 in, 2 out]
                              n412 = local write "SeqFreeErr"(w719) -> ()
                              n413 = local write "DevFreeErr"(w720) -> ()
                            }
                            frame #1 {
                              # "Play movie"
                              n414 = local read "DMD_trigger"() -> (w723:tag)
                              n415 = local read "DAQ Error"() -> (w722:errorcluster)
                              n416 = local read "Play Movie"() -> (w731:bool)
                              n417 = call-poly <vilib>:"DAQmx Create Virtual Channel.vi"("lines"=w723, "error in"=w722) -> ("task out"=w724:refnum<k21>, "error out"=w725:errorcluster)  [unwired: 3 in, 9 out]
                              n418 = call <vilib>:"DAQmx Start Task.vi"("task/channels in"=w724, "error in"=w725) -> ("task out"=w726:refnum<k21>, "error out"=w727:errorcluster)  [unwired: 12 out]
                              n419 = call-poly <vilib>:"DAQmx Write.vi"("task/channels in"=w726, "auto start"=TRUE, "data"=w731, "error in"=w727) -> ("task out"=w728:refnum<k21>, "error out"=w729:errorcluster)  [unwired: 9 in, 1 out]
                              n420 = call <vilib>:"DAQmx Clear Task.vi"("task in"=w728, "error in"=w729) -> ("error out"=w721:errorcluster)  [unwired: 13 out]
                              n421 = local write "DAQ Error"(w721) -> ()
                            }
                          }
                        }
                        frame True {
                          n422 = flat-sequence {
                            tunnel: w732 -> [w739]
                            frame #0 {
                              n423 = call "sub_load_DMD_mov_ext_trig.vi"("SequenceRepeats"=1, "binary mov path"=w739) -> ("SequID"=w736:u32, "DeviceID"=w737:u32, "DevInq1"=w735:errorcluster)
                              n424 = local write "DeviceID"(w737) -> ()
                              n425 = local write "SequID"(w736) -> ()
                              n426 = local write "ALP_Error"(w735) -> ()
                              n427 = property on="Image Registration" class="Bool (strict)"("DisabledEnum"=T5."Disabled and Grayed Out" ("Disabled")) -> ()  [unwired: 2 in, 2 out]
                              n428 = property on="All On" class="Bool (strict)"("DisabledEnum"=T5."Disabled and Grayed Out" ("Disabled")) -> ()  [unwired: 2 in, 2 out]
                            }
                            frame #1 {
                              # "Play movie"
                              n429 = local read "DMD_trigger"() -> (w742:tag)
                              n430 = local read "DAQ Error"() -> (w741:errorcluster)
                              n431 = local read "Play Movie"() -> (w750:bool)
                              n432 = call-poly <vilib>:"DAQmx Create Virtual Channel.vi"("lines"=w742, "error in"=w741) -> ("task out"=w743:refnum<k21>, "error out"=w744:errorcluster)  [unwired: 3 in, 9 out]
                              n433 = call <vilib>:"DAQmx Start Task.vi"("task/channels in"=w743, "error in"=w744) -> ("task out"=w745:refnum<k21>, "error out"=w746:errorcluster)  [unwired: 12 out]
                              n434 = call-poly <vilib>:"DAQmx Write.vi"("task/channels in"=w745, "auto start"=TRUE, "data"=w750, "error in"=w746) -> ("task out"=w747:refnum<k21>, "error out"=w748:errorcluster)  [unwired: 9 in, 1 out]
                              n435 = call <vilib>:"DAQmx Clear Task.vi"("task in"=w747, "error in"=w748) -> ("error out"=w740:errorcluster)  [unwired: 13 out]
                              n436 = local write "DAQ Error"(w740) -> ()
                            }
                          }
                        }
                      }
                    }
                    event "Contrast\nAdjust": Value Change {
                      n437 = event-data() -> ()  [unwired: 1 in, 1 out]
                      n438 = Unbundle("Contrast\nAdjust") -> (w757:i32, w756:i32)
                      n439 = Max & Min(x=w757, y=w756) -> (max(x,y)=w755:i32, min(x,y)=w754:i32)
                      n440 = property on="Image" class="IntGraph (strict)"("ZScale.Maximum"=w755, "ZScale.Minimum"=w754) -> ()  [unwired: 2 in, 2 out]
                      n441 = property on="Histogram" class="XYGraph (strict)"("XScale.Maximum"=w755, "XScale.Minimum"=w754) -> ()  [unwired: 2 in, 2 out]
                    }
                    event "473 signal", "473nm", "635nm": Value Change {
                      w768 = 0 items=["one channel for each line", "one channel for all lines"] ("line grouping")
                      n442 = event-data() -> ()  [unwired: 1 in, 1 out]
                      n443 = Select(t="473 signal", s="473nm", f=0.033) -> (s? t:f=w771:dbl)
                      n444 = local read "DAQ Error"() -> (w775:errorcluster)
                      n445 = call "subSetAnalogOut_cokecan.vi"("Error in (no error)"=w775, "AO value (0)"=w771, "AO line"="473nm line") -> ("Error out"=w763:errorcluster)  [unwired: 8 in]
                      n446 = call-poly <vilib>:"DAQmx Create Virtual Channel.vi"("lines"="635nm dig line", "line grouping"=w768, "error in"=w763) -> ("task out"=w770:refnum<k21>, "error out"=w769:errorcluster)  [unwired: 2 in, 9 out]
                      n447 = call <vilib>:"DAQmx Start Task.vi"("task/channels in"=w770, "error in"=w769) -> ("task out"=w767:refnum<k21>, "error out"=w766:errorcluster)  [unwired: 12 out]
                      n448 = call-poly <vilib>:"DAQmx Write.vi"("task/channels in"=w767, "auto start"=TRUE, "data"="635nm", "error in"=w766) -> ("task out"=w765:refnum<k21>, "error out"=w764:errorcluster)  [unwired: 10 out]
                      n449 = call <vilib>:"DAQmx Clear Task.vi"("task in"=w765, "error in"=w764) -> ("error out"=w761:errorcluster)  [unwired: 13 out]
                      n450 = local write "DAQ Error"(w761) -> ()
                    }
                    event "All On": Value Change {
                      n451 = event-data() -> ()  [unwired: 1 in, 1 out]
                      n452 = local read "All On"() -> (w782:bool)
                      n453 = case shown="False" w782 {
                        tunnel: path "C:/data/Lukas_data/all_on.bin" -> [_ w800]
                        frame False {
                          n454 = flat-sequence {
                            frame #0 {
                              n455 = local read "DeviceID"() -> (w786:u32)
                              n456 = local read "SequID"() -> (w785:u32)
                              n457 = call "sub_remove_DMD_mov.vi"("SequenceId"=w785, "DeviceId"=w786) -> ("SeqFreeErr"=w787:i32, "DevFreeErr"=w788:i32)
                              n458 = property on="Image Registration" class="Bool (strict)"("DisabledEnum"=T5."Enabled" ("Disabled")) -> ()  [unwired: 2 in, 2 out]
                              n459 = property on="Play Movie" class="Bool (strict)"("DisabledEnum"=T5."Enabled" ("Disabled")) -> ()  [unwired: 2 in, 2 out]
                              n460 = local write "SeqFreeErr"(w787) -> ()
                              n461 = local write "DevFreeErr"(w788) -> ()
                            }
                            frame #1 {
                              # "Play movie"
                              n462 = local read "DMD_trigger"() -> (w792:tag)
                              n463 = local read "DAQ Error"() -> (w791:errorcluster)
                              n464 = local read "All On"() -> (w789:bool)
                              n465 = call-poly <vilib>:"DAQmx Create Virtual Channel.vi"("lines"=w792, "error in"=w791) -> ("task out"=w793:refnum<k21>, "error out"=w794:errorcluster)  [unwired: 3 in, 9 out]
                              n466 = call <vilib>:"DAQmx Start Task.vi"("task/channels in"=w793, "error in"=w794) -> ("task out"=w795:refnum<k21>, "error out"=w796:errorcluster)  [unwired: 12 out]
                              n467 = call-poly <vilib>:"DAQmx Write.vi"("task/channels in"=w795, "auto start"=TRUE, "data"=w789, "error in"=w796) -> ("task out"=w797:refnum<k21>, "error out"=w798:errorcluster)  [unwired: 9 in, 1 out]
                              n468 = call <vilib>:"DAQmx Clear Task.vi"("task in"=w797, "error in"=w798) -> ("error out"=w790:errorcluster)  [unwired: 13 out]
                              n469 = local write "DAQ Error"(w790) -> ()
                            }
                          }
                        }
                        frame True {
                          n470 = flat-sequence {
                            tunnel: w800 -> [w807]
                            frame #0 {
                              n471 = call "sub_load_DMD_mov_ext_trig.vi"("SequenceRepeats"=1, "binary mov path"=w807) -> ("SequID"=w804:u32, "DeviceID"=w805:u32, "DevInq1"=w803:errorcluster)
                              n472 = property on="Image Registration" class="Bool (strict)"("DisabledEnum"=T5."Disabled and Grayed Out" ("Disabled")) -> ()  [unwired: 2 in, 2 out]
                              n473 = local write "DeviceID"(w805) -> ()
                              n474 = local write "SequID"(w804) -> ()
                              n475 = local write "ALP_Error"(w803) -> ()
                              n476 = property on="Play Movie" class="Bool (strict)"("DisabledEnum"=T5."Disabled and Grayed Out" ("Disabled")) -> ()  [unwired: 2 in, 2 out]
                            }
                            frame #1 {
                              # "Play movie"
                              n477 = local read "DMD_trigger"() -> (w811:tag)
                              n478 = local read "DAQ Error"() -> (w810:errorcluster)
                              n479 = local read "All On"() -> (w808:bool)
                              n480 = call-poly <vilib>:"DAQmx Create Virtual Channel.vi"("lines"=w811, "error in"=w810) -> ("task out"=w812:refnum<k21>, "error out"=w813:errorcluster)  [unwired: 3 in, 9 out]
                              n481 = call <vilib>:"DAQmx Start Task.vi"("task/channels in"=w812, "error in"=w813) -> ("task out"=w814:refnum<k21>, "error out"=w815:errorcluster)  [unwired: 12 out]
                              n482 = call-poly <vilib>:"DAQmx Write.vi"("task/channels in"=w814, "auto start"=TRUE, "data"=w808, "error in"=w815) -> ("task out"=w816:refnum<k21>, "error out"=w817:errorcluster)  [unwired: 9 in, 1 out]
                              n483 = call <vilib>:"DAQmx Clear Task.vi"("task in"=w816, "error in"=w817) -> ("error out"=w809:errorcluster)  [unwired: 13 out]
                              n484 = local write "DAQ Error"(w809) -> ()
                            }
                          }
                        }
                      }
                    }
                  }
                  n485 = local read "Enter Live Mode"() -> (w92:bool)
                  n486 = Wait (ms)(milliseconds to wait=u32 50) -> ()  [unwired: 1 out]
                }
                n487 = call <userlib>:"tm_stopcapture.vi"("error in (no error)"=w73, "Handle in"=w72) -> ("error out"=w74:errorcluster, "Handle out"=w75:u32)  [unwired: 8 in]
                n488 = call <userlib>:"tm_unpreparecapture.vi"("error in (no error)"=w74, "Handle in"=w75) -> ("error out"=w71:errorcluster)  [unwired: 8 in, 1 out]
                n489 = local write "Camera Error"(w71) -> ()
              }
            }
          }
        }
      }
    }
    frame #2 {
      n490 = local read "Camera Error"() -> (w825:errorcluster)
      n491 = local read "Image Registration"() -> (w823:bool)
      n492 = local read "Play Movie"() -> (w822:bool)
      n493 = local read "All On"() -> (w820:bool)
      n494 = call <userlib>:"tm_closecamera.vi"("error in (no error)"=w825, "Handle in"=u32 0) -> ("error out"=w827:errorcluster)  [unwired: 9 in]
      n495 = call <userlib>:"tm_deinitialize.vi"("error in (no error)"=w827) -> ("error out"=w824:errorcluster)  [unwired: 10 in]
      n496 = Or(x=w823, y=w822) -> (x .or. y?=w821:bool)
      n497 = local write "Camera Error"(w824) -> ()
      n498 = Or(x=w821, y=w820) -> (x .or. y?=w819:bool)
      n499 = case shown="True" w819 {
        frame False {
        }
        frame True {
          # "Play movie"
          n500 = local read "DeviceID"() -> (w840:u32)
          n501 = local read "SequID"() -> (w839:u32)
          n502 = call "sub_remove_DMD_mov.vi"("SequenceId"=w839, "DeviceId"=w840) -> ("SeqFreeErr"=w841:i32, "DevFreeErr"=w842:i32)
          n503 = local write "SeqFreeErr"(w841) -> ()
          n504 = local write "DevFreeErr"(w842) -> ()
          n505 = local read "DMD_trigger"() -> (w831:tag)
          n506 = local read "DAQ Error"() -> (w830:errorcluster)
          n507 = call-poly <vilib>:"DAQmx Create Virtual Channel.vi"("lines"=w831, "error in"=w830) -> ("task out"=w832:refnum<k21>, "error out"=w833:errorcluster)  [unwired: 3 in, 9 out]
          n508 = call <vilib>:"DAQmx Start Task.vi"("task/channels in"=w832, "error in"=w833) -> ("task out"=w834:refnum<k21>, "error out"=w835:errorcluster)  [unwired: 12 out]
          n509 = call-poly <vilib>:"DAQmx Write.vi"("task/channels in"=w834, "auto start"=TRUE, "data"=FALSE ("auto start"), "error in"=w835) -> ("task out"=w836:refnum<k21>, "error out"=w837:errorcluster)  [unwired: 9 in, 1 out]
          n510 = call <vilib>:"DAQmx Clear Task.vi"("task in"=w836, "error in"=w837) -> ("error out"=w829:errorcluster)  [unwired: 13 out]
          n511 = local write "DAQ Error"(w829) -> ()
        }
      }
    }
  }
